vi "出厂检测.vi"() -> ()   [LabVIEW 2016]
uses:
  Ctl/AllSeting.ctl
  Ctl/Option.ctl
  controls/P2Judge QueueCtl.ctl
  <vilib>/vision/Image Controls.llb/IMAQ Image.ctl
panel:
  out "Array":u16[][](array[numeric])
  out "before substring":string
  out "Intensity Graph":u16[][](graph)
  out "Image":T1(plugin-control)
  in  "Button - Exit":bool
  in  "Button - Option":bool caption="Blank Button"
  in  "Button - Searchdata":bool caption="Blank Button"
  out "process":string
  in  "选项卡控件":enum32{"采集信息", "模组参数", "调试信息"}(tab)
  out "Tempparm_D合格？":bool
  out "NUC-T_D合格？":bool
  out "BT_D合格？":bool
  out "KT_D合格？":bool
  out "Tempparm合格？":bool
  out "NUC-T合格?":bool
  out "BT合格？":bool
  out "KT合格？":bool
  out "Tempparm一致性":bool
  out "NUC-T一致性":bool
  out "BT一致性":bool
  out "KT一致性":bool
  in  "固件版本":string
  in  "手动打印二维码":bool caption="Blank Button"
  in  "物料号":string="76"
  in  "型号":string(combo)="C"
  in  "打印列":u16(ring) items=["第一列", "第二列", "第三列", "第四列", "第五列"]
  in  "SN":string
  in  "PN":string
  out "盲元合格":bool
  in  "ID":string
  out "盲元数":dbl
  out "切换增益成功":bool
  out "state":string
  out "温度差值1":dbl
  out "读取温度1":dbl
  out "黑体设定温度1":dbl
  out "高增益温度误差在范围内":bool
  out "温度差值2":dbl
  out "读取温度2":dbl
  out "黑体设定温度2":dbl
  out "低增益温度误差在范围内":bool
  out "二维码信息":string
  out "当前流水号":string
  in  "当前增益模式":enum16{"低增益", "高增益"}(ring)
  out "近标靶是否合格":bool
  out "远标靶是否合格":bool
  out "近调焦垂直清晰度":dbl caption="垂直清晰度"
  out "近调焦水平清晰度":dbl caption="水平清晰度"
  out "远调焦水平清晰度":dbl caption="水平清晰度"
  out "远调焦垂直清晰度":dbl caption="垂直清晰度"
  out "低增益数据合格？":bool
  out "高增益数据合格？":bool
  out "Tempparam_Default":u8[](graph)
  out "NUC-T_Default":u16[](graph)
  out "BT_Default":i16[](graph)
  out "KT_Default":u16[](graph)
  out "Tempparam":u8[](graph)
  out "NUC-T":u16[](graph)
  out "BT":i16[](graph)
  out "KT":u16[](graph)
  in  "出图":bool
  out "Caldata.Fps":u16
  out "source path out":path
  out "调焦数值min":i32
  out "标定前盲元":dbl
  out "盲元表":dbl[][](array[numeric])
  out "调焦数值min2":i32
  out "检查锅盖竖纹是否合格":bool
  out "分辨率":string
  out "agc":u16
  in  "写入配置":bool caption="Blank Button"
  in  "打开AGC":bool caption="Blank Button"
  in  "读取盲元数":bool caption="Blank Button"
  in  "流水号归零":bool caption="Blank Button"
  in  "读ID":bool caption="Blank Button"
  in  "打快门":bool caption="Blank Button"
  out "参数存储地址":path
  out "Numeric":dbl format="%#_13g"
  in  "Button - start":bool caption="Blank Button"
  in  "完成":bool caption="Blank Button"
  # "在存储地址放入模板"
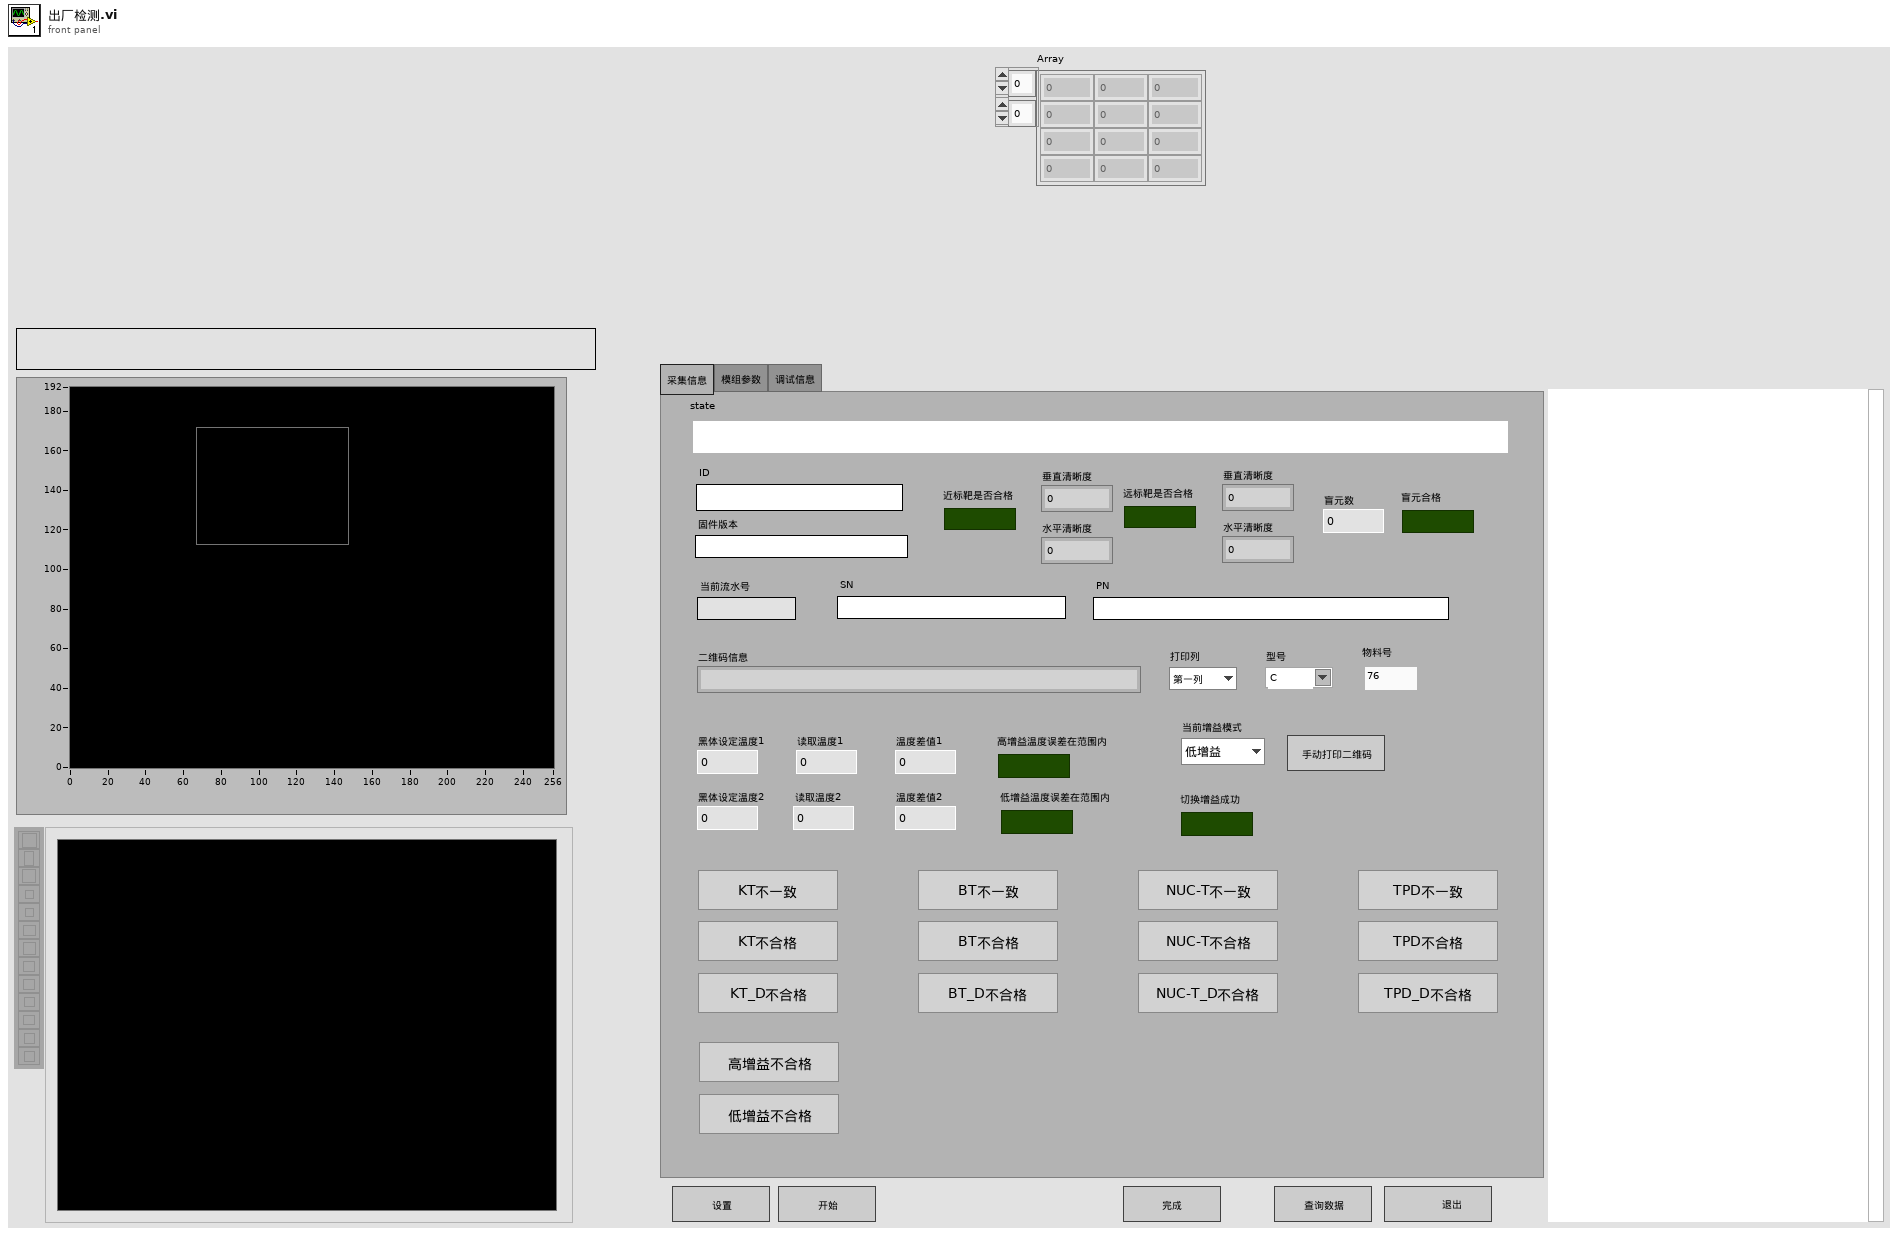
[diagram p1: front panel]
types:
  T1 = typedef "IMAQ Image.ctl" = refnum<image>
  T2 = typedef "AllSeting.ctl" = cluster{"Caldata":T3}
  T3 = typedef "Option.ctl" = cluster{"分辨率":string, "Fps":u16, "工单号":string, "操作人":string, "增益模式":enum16{"高低增益切换", "高增益"}, "黑体设定温度1":dbl, "温差范围1":dbl, "出图到测温等待时间":dbl, "调焦数值min":i32, "盲元阈值":dbl, "盲元采样帧数":u16, "调焦数值min2":i32, "黑体设定温度2":dbl, "温差范围2":dbl, "ID选择":enum16{"旧ID", "新ID"}, "快门时间间隔设置":cluster{"快门第一次延时时间":u16, "快门第二次延时时间":u16, "切换增益后快门第一次延时时间":u16, "切换增益后快门第二次延时时间":u16}, "产品名":string, "镜头":string, "测温功能":string, "产品料号":string, "打印机VISA":refnum<visa-resource-name>, "焦距选择":enum32{"Radio Selection 1", "Radio Selection 2", "Radio Selection 3"}, "工位":string, "服务器保存地址":path}
  T4 = typedef "P2Judge QueueCtl.ctl" = enum16{"Main", "Device", "Picture"}
  T5 = typedef "QueueModeCtl.ctl" = enum16{"<no operate>", "Send", "Send(head)", "Flush", "Destory", "Send>All", "Send>All(head)", "Flush All", "Destory All"}
  T6 = cluster{"CalData":path, "Datasave":path, "Data":path}
  T7 = enum32{"Radio Selection 1", "Radio Selection 2", "Radio Selection 3"}
  T8 = cluster{"快门第一次延时时间":u16, "快门第二次延时时间":u16, "切换增益后快门第一次延时时间":u16, "切换增益后快门第二次延时时间":u16}
  T9 = typedef "LVPointDoubleTypeDef.ctl" = cluster{"Cursor X":dbl, "Cursor Y":dbl}
  T10 = enum32{"invalid app kind", "Development System", "Run Time System", "Student Edition", "Embedded LabVIEW", "Evaluation", "Custom"}
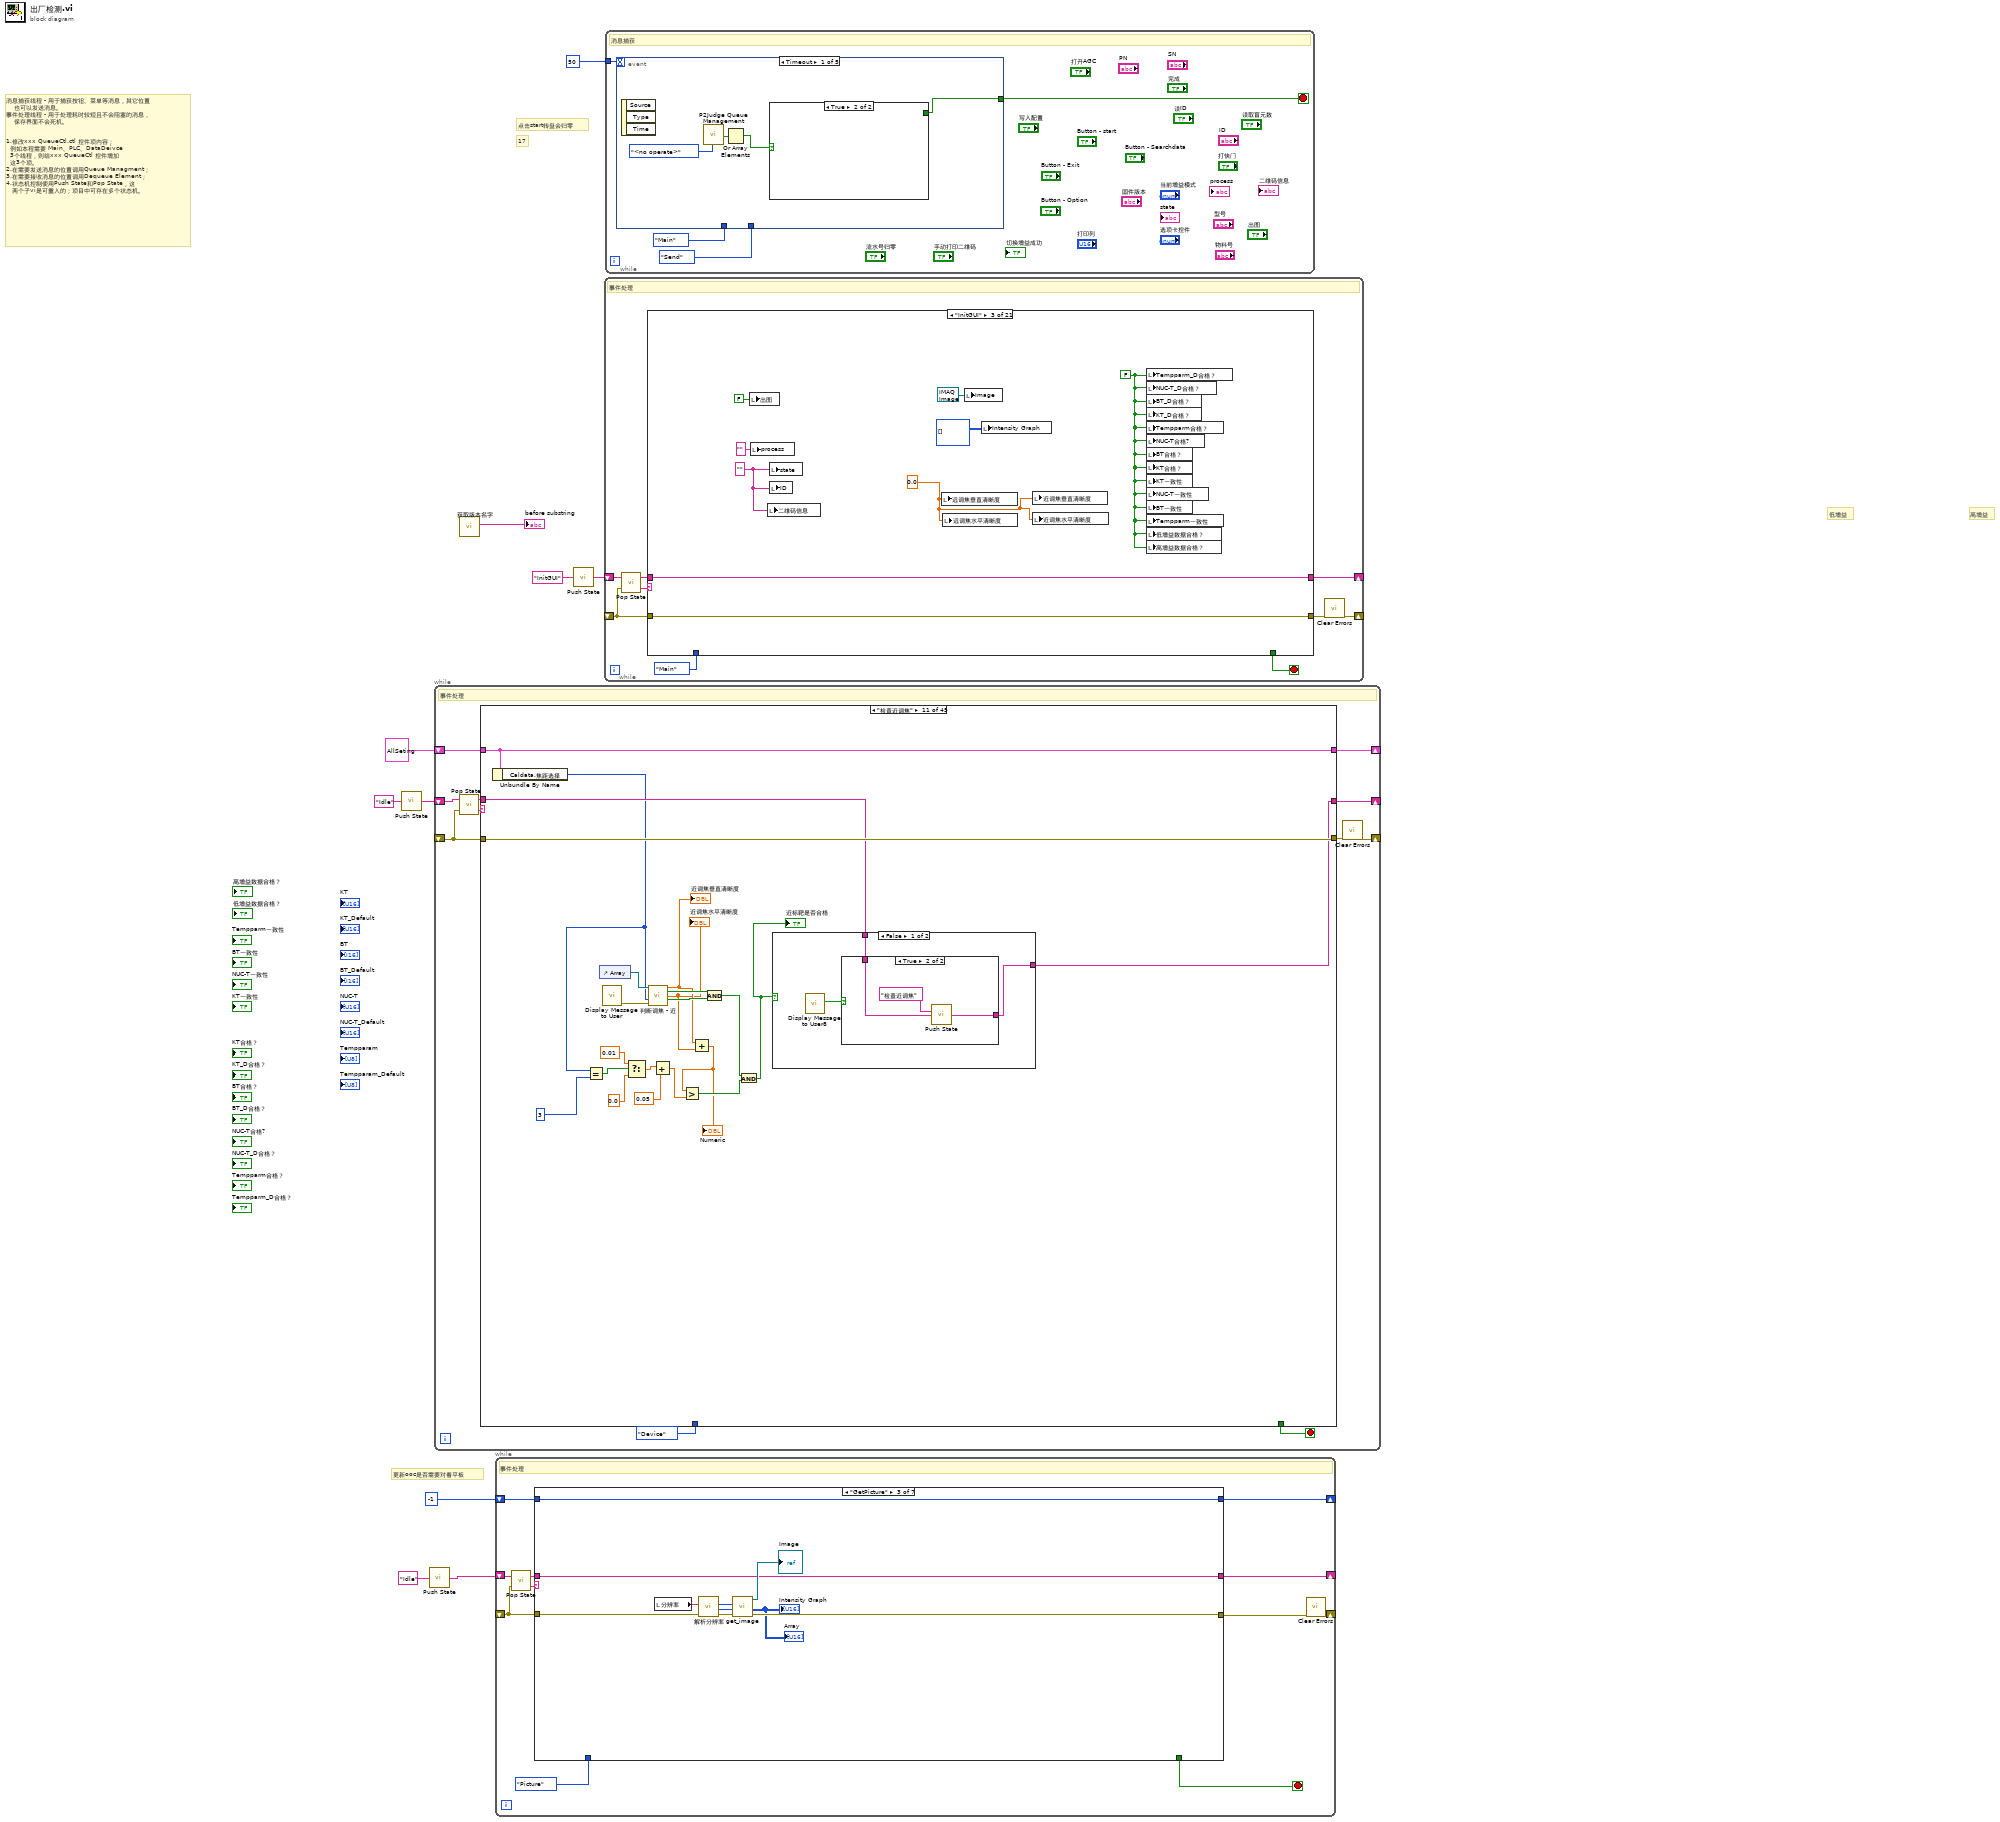
[diagram p0: block diagram]
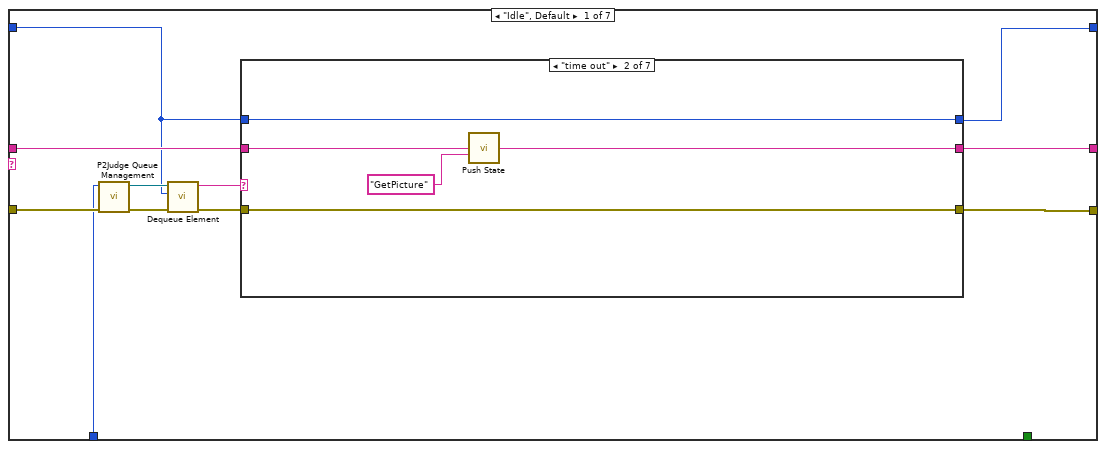
[diagram p2: hidden frame]
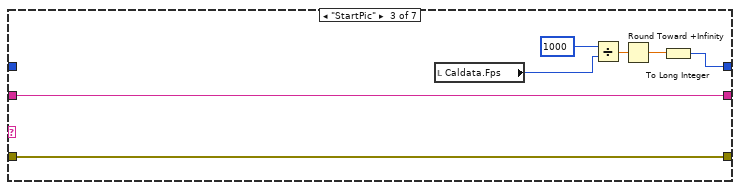
[diagram p4: hidden frame]
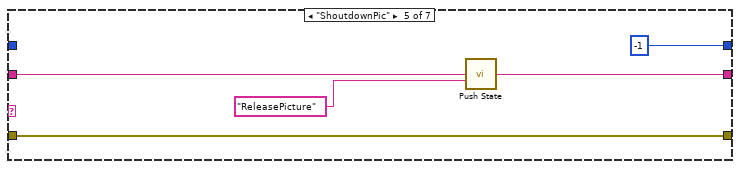
[diagram p6: hidden frame]
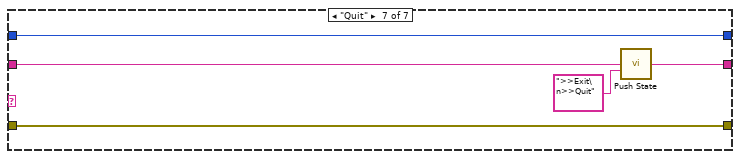
[diagram p8: hidden frame]
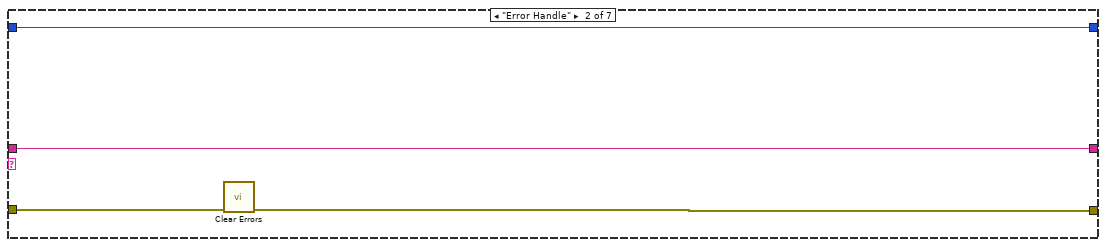
[diagram p9: hidden frame]
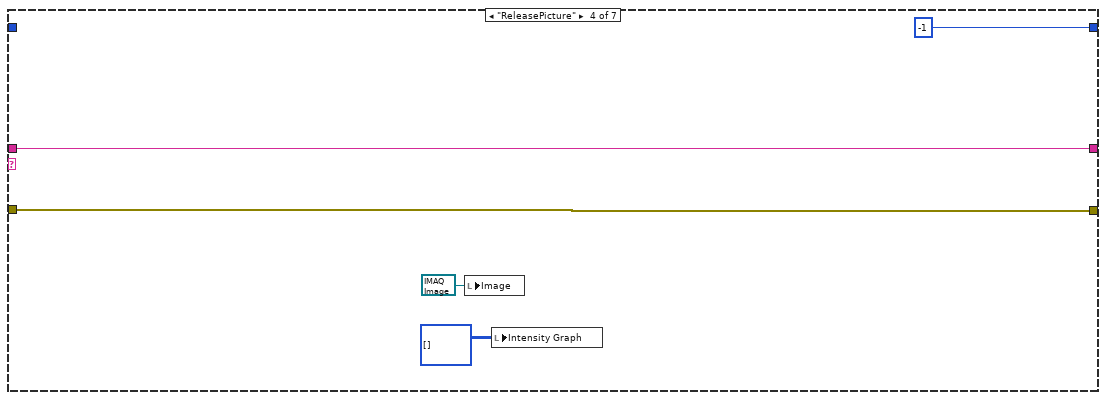
[diagram p10: hidden frame]
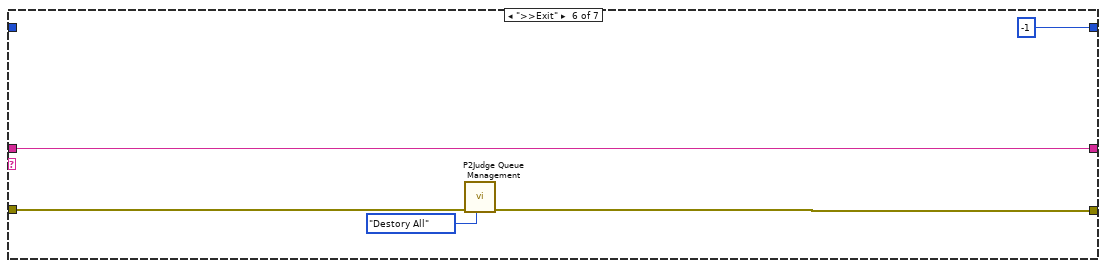
[diagram p12: hidden frame]
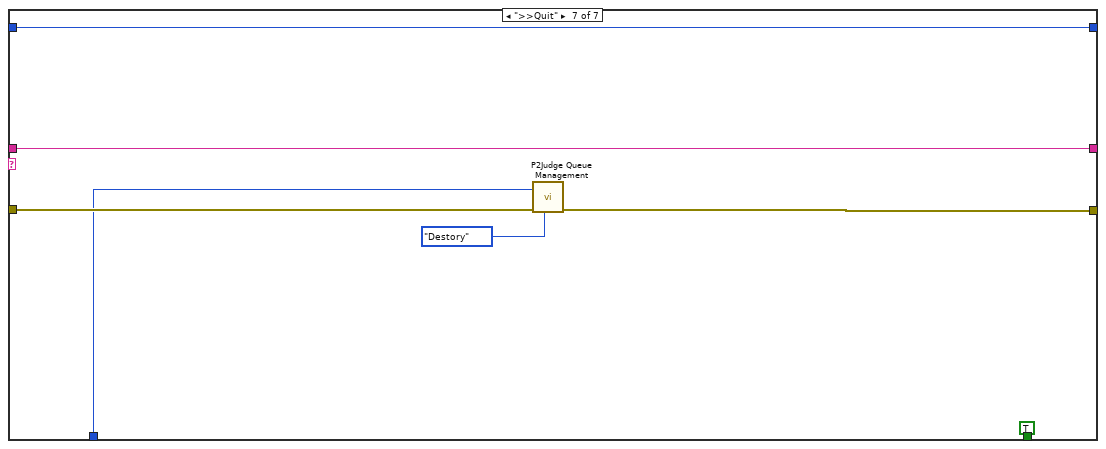
[diagram p13: hidden frame]
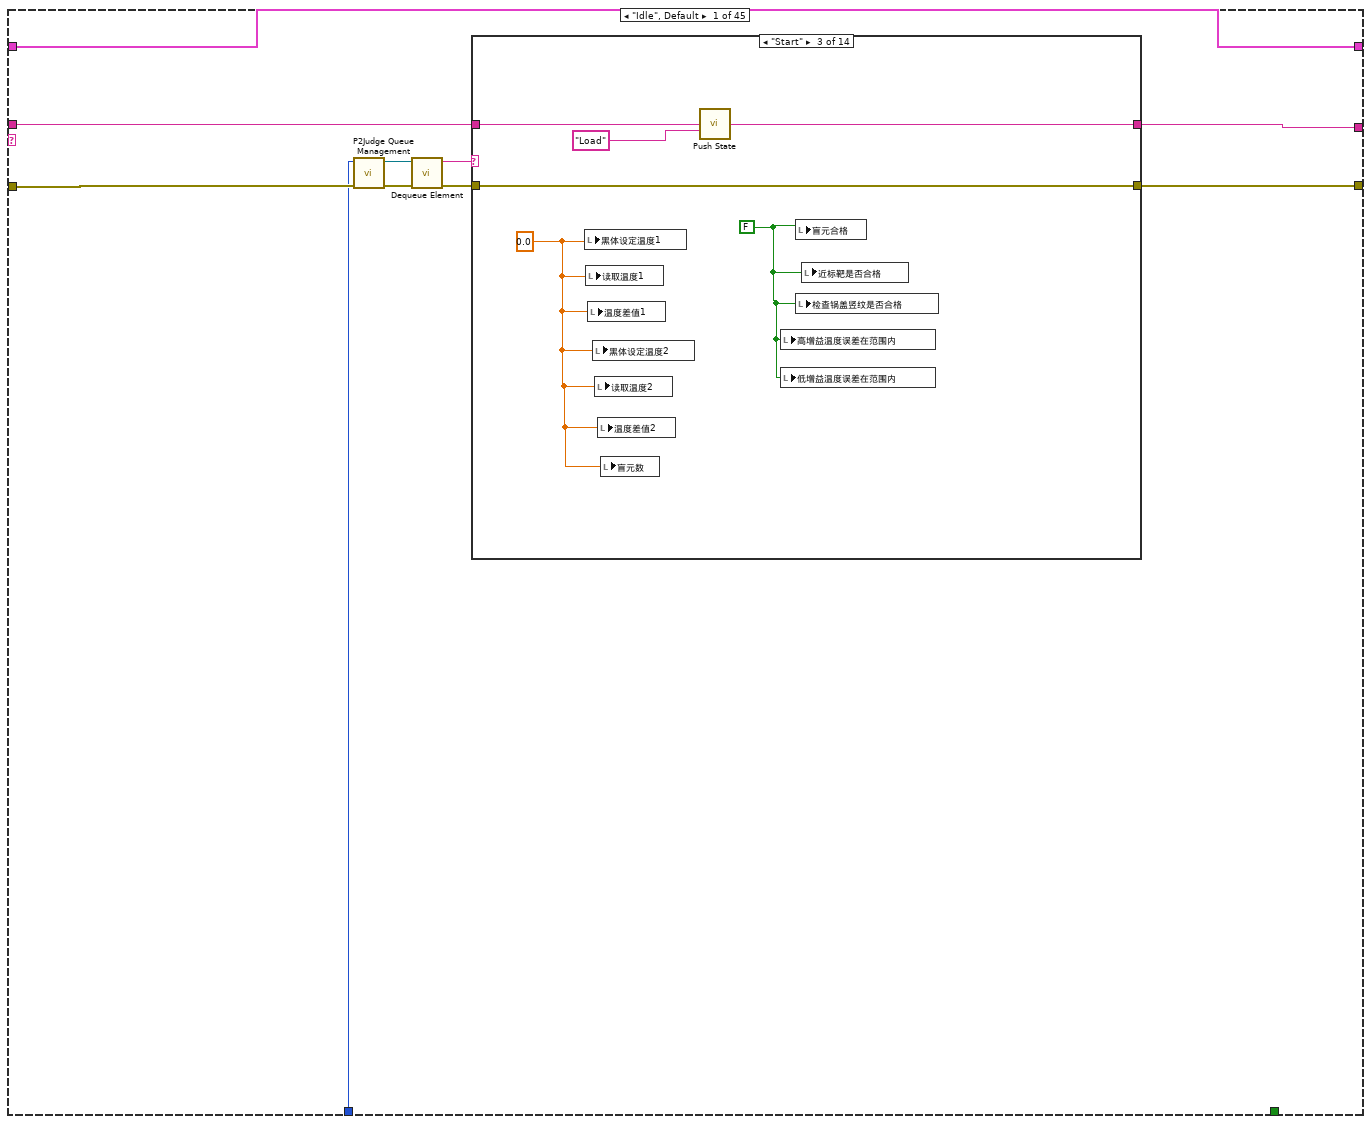
[diagram p14: hidden frame]
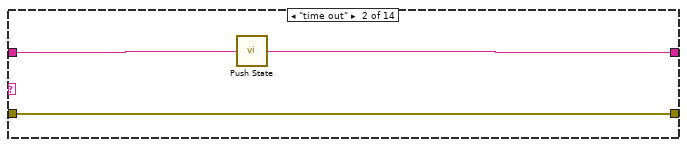
[diagram p16: hidden frame]
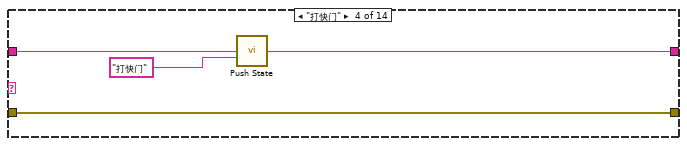
[diagram p17: hidden frame]
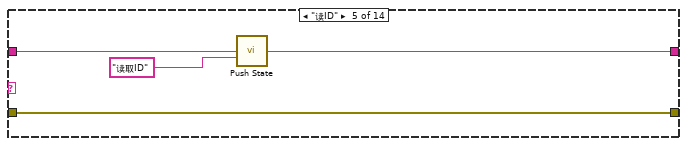
[diagram p18: hidden frame]
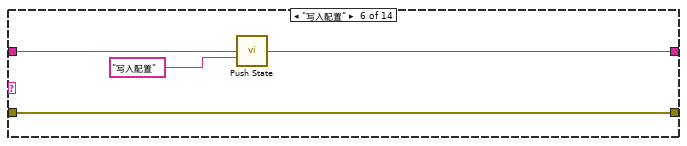
[diagram p19: hidden frame]
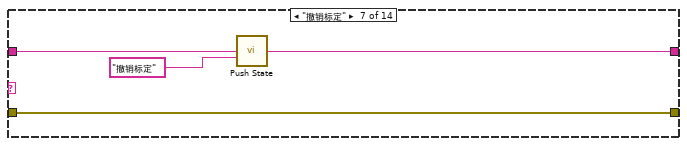
[diagram p20: hidden frame]
diagram:
  # "高增益"
  # "低增益"
  # "17"
  # "更新ooc是否需要对着平板"
  # "点击start转盘会归零"
  # "消息捕获线程 - 用于捕获按钮、菜单等消息，其它位置\n    也可以发送消息。\n事件处理线程 - 用于处理耗时较短且不会阻塞的消息，\n    保存界面不会死机。\n\n\n1.修改xxx QueueCtl.ctl 控件项内容；\n  例如本程需要 Main、PLC、DataDeivce\n  3个线程，则给xxx QueueCtl 控件增加\n  这3个项。\n2.在需要发送消息的位置调用Queue Managment；\n3.在需要接收消息的位置调用Dequeue Element；\n4.状态机控制使用Push State和Pop State，这\n   两个子vi是可重入的；项目中可存在多个状态机。"
  n1 = call "Push State.vi"("States In"="Idle") -> ("States Out"=w6:string)  [unwired: 14 in]
  n2 = call "Push State.vi"("States In"="Idle") -> ("States Out"=w3:string)  [unwired: 14 in]
  n3 = while {
    shift-right: [w19] -> _
    shift-left: w6 -> [w21]
    shift-right: [w11] -> _
    shift-left: _ -> [w17]
    shift-right: [w14] -> _
    shift-left: T2 {"Caldata"={"分辨率"="", "Fps"=0, "工单号"="", "操作人"="", "增益模式"=enum."高低增益切换", "黑体设定温度1"=0.0, "温差范围1"=0.0, "出图到测温等待时间"=0.0, "调焦数值min"=0, "盲元阈值"=0.0, "盲元采样帧数"=0, "调焦数值min2"=0, "黑体设定温度2"=0.0, "温差范围2"=0.0, "ID选择"=enum."旧ID", "快门时间间隔设置"={"快门第一次延时时间"=200, "快门第二次延时时间"=200, "切换增益后快门第一次延时时间"=200, "切换增益后快门第二次延时时间"=200}, "产品名"="Tiny1-C", "镜头"="02011X", "测温功能"="WR", "产品料号"="", "打印机VISA"="", "焦距选择"=enum."Radio Selection 1", "工位"="0001", "服务器保存地址"=path ""}} ("all setting") -> [w13]
    stop <- w16 stop-if-true
    # "事件处理"
    n4 = call "Pop State.vi"("error in (no error)"=w17, "Pre States"=w21) -> ("New State"=w20:string, "Remaining States"=w18:string)
    n5 = case shown="\"检查近调焦\"" w20 {
      tunnel: [w25 w88 w91 w112 w141 w171 w205 w232 w252 w265 w292 w333 w350 w358 w400 w438 w453 w484 w506 w525 w574 w625 w650 w678 w694 w706 w766 w786 w881 w1045 w1080 w1102 w1109 w1145 w1167 w1244 w1303 w1350 w1383 w1411 w1413 w1437 w1447 w1475 w1482] -> w19
      tunnel: w18 -> [w24 w88 w91 _ w143 w172 w207 w234 w252 w265 w291 w332 w350 w355 w401 w439 w454 w485 w507 w526 w575 w626 w651 w675 w694 w706 w767 w788 w882 w1046 w1081 w1102 w1110 w1145 w1168 w1245 w1304 w1351 w1384 w1411 w1414 w1437 w1448 w1475 w1482]
      tunnel: [w28 w86 w90 w117 w144 w164 w206 w233 w253 w266 w295 w336 w347 w359 w402 w440 w455 w486 w508 w527 w576 w627 w652 w679 w695 w705 w768 w846 w880 w1047 w1082 w1101 w1111 w1140 w1169 w1246 w1288 w1334 w1382 w1409 w1415 w1438 w1449 w1473 w1478] -> w12
      tunnel: w17 -> [w31 w87 w90 w122 w140 w167 w211 w238 w257 w270 w295 w336 w348 w368 w395 w433 w460 w488 w510 w528 w577 w628 w653 w680 w700 w708 w771 w847 w941 w1048 w1085 w1103 w1116 w1146 w1173 w1248 w1305 w1352 w1388 w1410 w1419 w1441 w1453 w1474 w1479]
      tunnel: [_ _ _ _ _ _ _ _ _ _ _ _ _ _ _ _ _ _ _ _ _ _ _ _ _ _ _ _ _ _ _ _ _ _ _ _ _ _ _ _ _ _ _ _ TRUE] -> w16
      tunnel: P2Judge_QueueCtl."Device" ("Queue Index") -> [w23 _ _ _ _ _ _ _ _ _ _ _ _ _ _ _ _ _ _ _ _ _ _ _ _ _ _ _ _ _ _ _ _ _ _ _ _ _ _ _ _ _ _ _ w1477]
      tunnel: [w22 w85 w89 w114 w130 w163 w215 w239 w251 w264 w289 w330 w349 w370 w403 w441 w465 w475 w503 w524 w573 w624 w649 w677 w699 w707 w776 w844 w940 w1040 w1090 w1108 w1121 w1139 w1158 w1242 w1299 w1346 w1393 w1408 w1412 w1440 w1451 w1471 w1476] -> w14
      tunnel: w13 -> [w22 w85 w89 w113 w130 w163 w215 w239 w251 w264 w289 w330 w349 w370 w403 w441 w465 w475 w503 w524 w573 w624 w649 w677 w699 w707 w776 w844 w940 w1040 w1090 w1108 w1121 w1139 w1158 w1242 w1299 w1346 w1393 w1408 w1412 w1440 w1451 w1471 w1476]
      frame "Idle", Default {
        n6 = call "P2Judge Queue Management.vi"("error in"=w31, "Queue Index"=w23) -> ("error out"=w30:errorcluster, "Queue"=w29:refnum<queue>)  [unwired: 7 in, 1 out]
        n7 = call "Dequeue Element.vi"("error in"=w30, "Queue"=w29) -> ("error out"=w27:errorcluster, "Command"=w26:string)  [unwired: 7 in, 1 out]
        n8 = case shown="\"Start\"" w26 {
          tunnel: [w33 w36 w42 w46 w50 w54 w58 w62 w66 w70 w74 w78 w80 w84] -> w28
          tunnel: w27 -> [w33 w36 w42 w46 w50 w54 w58 w62 w66 w70 w74 w78 w80 w84]
          tunnel: [w32 w34 w40 w44 w48 w52 w56 w60 w64 w68 w72 w76 w79 w82] -> w25
          tunnel: w24 -> [w32 w35 w41 w45 w49 w53 w57 w61 w65 w69 w73 w77 w79 w83]
          frame Default {
          }
          frame "time out" {
            n9 = call "Push State.vi"("States In"=w35) -> ("States Out"=w34:string)  [unwired: 14 in]
          }
          frame "Start" {
            w38 = 0.0
            w37 = FALSE
            n10 = local write "黑体设定温度1"(w38) -> ()
            n11 = local write "读取温度1"(w38) -> ()
            n12 = local write "温度差值1"(w38) -> ()
            n13 = local write "黑体设定温度2"(w38) -> ()
            n14 = local write "读取温度2"(w38) -> ()
            n15 = local write "温度差值2"(w38) -> ()
            n16 = local write "盲元数"(w38) -> ()
            n17 = call "Push State.vi"("States In"=w41, "States End"="Load") -> ("States Out"=w40:string)  [unwired: 13 in]
            n18 = local write "高增益温度误差在范围内"(w37) -> ()
            n19 = local write "低增益温度误差在范围内"(w37) -> ()
            n20 = local write "盲元合格"(w37) -> ()
            n21 = local write "检查锅盖竖纹是否合格"(w37) -> ()
            n22 = local write "近标靶是否合格"(w37) -> ()
          }
          frame "打快门" {
            n23 = call "Push State.vi"("States In"=w45, "States End"="打快门") -> ("States Out"=w44:string)  [unwired: 13 in]
          }
          frame "读ID" {
            n24 = call "Push State.vi"("States In"=w49, "States End"="读取ID") -> ("States Out"=w48:string)  [unwired: 13 in]
          }
          frame "写入配置" {
            n25 = call "Push State.vi"("States In"=w53, "States End"="写入配置") -> ("States Out"=w52:string)  [unwired: 13 in]
          }
          frame "撤销标定" {
            n26 = call "Push State.vi"("States In"=w57, "States End"="撤销标定") -> ("States Out"=w56:string)  [unwired: 13 in]
          }
          frame "打开AGC" {
            n27 = call "Push State.vi"("States In"=w61, "States End"="打开AGC") -> ("States Out"=w60:string)  [unwired: 13 in]
          }
          frame "打印二维码" {
            n28 = call "Push State.vi"("States In"=w65, "States End"="打印二维码") -> ("States Out"=w64:string)  [unwired: 13 in]
          }
          frame "流水号归零" {
            n29 = call "Push State.vi"("States In"=w69, "States End"="流水号归零") -> ("States Out"=w68:string)  [unwired: 13 in]
          }
          frame "读取盲元数" {
            n30 = call "Push State.vi"("States In"=w73, "States End"="读取盲元数") -> ("States Out"=w72:string)  [unwired: 13 in]
          }
          frame "完成" {
            n31 = call "Push State.vi"("States In"=w77, "States End"="保存出厂检测数据\n关闭相机") -> ("States Out"=w76:string)  [unwired: 13 in]
          }
          frame "error" {
          }
          frame "Quit" {
            n32 = call "Push State.vi"("States In"=w83, "States End"=">>Exit\n>>Quit" ("Remaining States")) -> ("States Out"=w82:string)  [unwired: 13 in]
          }
        }
      }
      frame "Error Handle" {
        n33 = call <vilib>:"Clear Errors.vi"("error in (no error)"=w87) -> ("error out"=w86:errorcluster)  [unwired: 5 in, 1 out]
      }
      frame ">>Init" {
      }
      frame "Load" {
        w92 = FALSE ("Tempparm_D合格？")
        w124 = "下载配置" ("state")
        n34 = local read "process"() -> (w125:string)
        n35 = property on="state" class="Str"(error in=w122, "Value"=w124) -> (error out=w126:errorcluster)  [unwired: 1 in, 1 out]
        n36 = call "process.vi"("error in"=w126, "state"=w124, "process in"=w125) -> ("error out"=w121:errorcluster, "process out"=w123:string)  [unwired: 7 in]
        n37 = local write "Tempparm_D合格？"(w92) -> ()
        n38 = local write "NUC-T_D合格？"(w92) -> ()
        n39 = local write "BT_D合格？"(w92) -> ()
        n40 = local write "KT_D合格？"(w92) -> ()
        n41 = local write "Tempparm合格？"(w92) -> ()
        n42 = local write "NUC-T合格?"(w92) -> ()
        n43 = local write "BT合格？"(w92) -> ()
        n44 = local write "KT合格？"(w92) -> ()
        n45 = local write "KT一致性"(w92) -> ()
        n46 = local write "NUC-T一致性"(w92) -> ()
        n47 = local write "BT一致性"(w92) -> ()
        n48 = local write "Tempparm一致性"(w92) -> ()
        n49 = local write "低增益数据合格？"(w92) -> ()
        n50 = local write "高增益数据合格？"(w92) -> ()
        n51 = call "Path.vi"() -> ("path"=w120:T6)  [unwired: 9 in]
        n52 = local write "process"(w123) -> ()
        n53 = Unbundle By Name(w120) -> ("CalData"=w119:path)
        n54 = call "Path.vi"() -> ()  [unwired: 9 in, 1 out]
        n55 = call "loadorsave_Option.vi"("save?"=FALSE, "error in"=w121, "Path in"=w119) -> ("error out"=w118:errorcluster, "Caldata out"=w115:T3)  [unwired: 6 in, 1 out]
        n56 = Unbundle By Name(w115) -> ("调焦数值min2"=→"调焦数值min2":i32, "调焦数值min"=→"调焦数值min":i32, "工单号"=w116:string, "增益模式"=w107:enum16{"高低增益切换", "高增益"}, "分辨率"=w100:string, "服务器保存地址"=w94:path)
        "分辨率" <- w100
        n57 = case shown="\"高低增益切换\", Default" w107 {
          tunnel: ["打开相机\n计算流水号\n读取ID\n读取固件版本\n关闭AGC\n关闭自动快门\n切换出图为SNR\n切换低增益\n出图到测温等待时间\n打快门\n读取低增益温度\n切换高增益\n出图到测温等待时间\n打快门\n读取高增益温度\n打快门\n检查近调焦\n检查远调焦\n检查锅盖竖纹\n打快门\n读取标定盲元\n打开自动快门\n绑定ID\n写入SN\n写入PN\n读取SNPN\n打开AGC\n保存数据\n生成出厂配置\n检查模组高增益参数\n检查模组低增益参数\n打印二维码\n出厂检完成" "打开相机\n计算流水号\n读取ID\n读取固件版本\n读取SNPN\n关闭AGC\n关闭自动快门\n切换出图为SNR\n切换高增益\n出图到测温等待时间\n打快门\n读取高增益温度\n打快门\n检查近调焦\n检查远调焦\n检查锅盖竖纹\n打快门\n读取标定盲元\n打开自动快门\n绑定ID\n写入SN\n写入PN\n读取SNPN\n打开AGC\n保存数据\n生成出厂配置\n检查模组高增益参数\n打印二维码\n出厂检完成"] -> w112
          frame "高低增益切换", Default {
          }
          frame "高增益" {
          }
        }
        n58 = Equal?(x=w100, y="256*192") -> (x = y?=w96:bool)
        n59 = Select(t="Tiny1Cflash.xlsx", s=w96, f="Tiny1Cflash小分辨率.xlsx") -> (s? t:f=w95:string)
        n60 = call "复制模板.vi"("error in"=w118, "服务器地址"=w94, "工单号"=w116) -> ("error out"=w109:errorcluster, "参数存储地址"=→"参数存储地址":path, "source path out"=→"source path out":path)  [unwired: 6 in]
        n61 = call "Path.vi"() -> ("path"=w106:T6)  [unwired: 9 in]
        n62 = Unbundle By Name(w106) -> ("Data"=w105:path)
        n63 = Build Path(base path=w105, name or relative path=w95) -> (appended path=w104:path)
        n64 = call "Read_Address_Map.vi"("file path"=w104) -> ("error out"=w103:errorcluster, "all rows"=w102:string[][])  [unwired: 9 in]
        n65 = Bundle By Name(cluster=w113, "Caldata"=w115) -> (w114:T2)
        n66 = call "2DStrArrayToEle.vi"("Mothed"=enum16{"init", "Get", "Set", "Close"}."Set", "error in"=w103, "all rows"=w102) -> ()  [unwired: 5 in, 4 out]
        n67 = call <vilib>:"Clear Errors.vi"("error in (no error)"=w109) -> ("error out"=w117:errorcluster)  [unwired: 5 in, 1 out]
      }
      frame "打开相机" {
        w138 = "打开相机" ("state")
        n68 = local read "process"() -> (w137:string)
        n69 = property on="state" class="Str"(error in=w140, "Value"=w138) -> (error out=w136:errorcluster)  [unwired: 1 in, 1 out]
        n70 = call "process.vi"("error in"=w136, "state"=w138, "process in"=w137) -> ("error out"=w135:errorcluster, "process out"=w139:string)  [unwired: 7 in]
        n71 = local write "process"(w139) -> ()
        n72 = Unbundle By Name(w130) -> ("Caldata.分辨率"=w134:string, "Caldata.Fps"=w133:u16)
        "Caldata.Fps" <- w133
        n73 = call "打开相机.vi"("error in"=w135, "FPS"=w133, "分辨率"=w134) -> ("error out"=w131:errorcluster, "result"=w132:bool)  [unwired: 6 in, 1 out]
        n74 = case shown="True" w132 {
          tunnel: ["操作失败关闭相机" w150] -> w142
          tunnel: w131 -> [w145 w149]
          tunnel: [w145 w147] -> w144
          tunnel: w143 -> [_ w150]
          frame False {
          }
          frame True {
            n75 = property on="出图" class="Bool (strict)"(error in=w149, "Val(Sgnl)"=TRUE ("Value (Signaling)")) -> (error out=w147:errorcluster)  [unwired: 1 in, 1 out]
          }
        }
        n76 = call "Push State.vi"("States In"=w142) -> ("States Out"=w141:string)  [unwired: 14 in]
      }
      frame "读取ID" {
        w170 = "读取ID" ("state")
        w176 = "_"
        n77 = local read "process"() -> (w169:string)
        n78 = property on="state" class="Str"(error in=w167, "Value"=w170) -> (error out=w168:errorcluster)  [unwired: 1 in, 1 out]
        n79 = call "process.vi"("error in"=w168, "state"=w170, "process in"=w169) -> ("error out"=w166:errorcluster, "process out"=w165:string)  [unwired: 7 in]
        n80 = local write "process"(w165) -> ()
        n81 = call "ReadID.vi"("error in"=w166) -> ("error out"=w173:errorcluster, "data out"=w189:u8[], "return"=w175:i32)  [unwired: 8 in]
        n82 = Index Array(array=w189) -> (element #1=w188:u8, element #2=w187:u8, element #3=w186:u8, element #4=w185:u8, element #5=w184:u8, element #6=w183:u8, element #7=w162:u8, element #8=w161:u8, element #9=w160:u8, element #10=w159:u8)  [unwired: 10 in]
        n83 = Join Numbers(hi=w160, lo=w159) -> ((hi.lo)=w157:u16)
        n84 = Join Numbers(hi=w162, lo=w161) -> ((hi.lo)=w158:u16)
        n85 = Join Numbers(hi=w188, lo=w187) -> ((hi.lo)=w182:u16)
        n86 = Join Numbers(hi=w186, lo=w185) -> ((hi.lo)=w181:u16)
        n87 = Join Numbers(hi=w184, lo=w183) -> ((hi.lo)=w180:u16)
        n88 = Join Numbers(hi=w158, lo=w157) -> ((hi.lo)=w156:u32)
        n89 = Number To Decimal String(number=w156) -> (decimal integer string=w153:string)  [unwired: 1 in]
        n90 = Number To Decimal String(number=w180) -> (decimal integer string=w177:string)  [unwired: 1 in]
        n91 = Number To Decimal String(number=w182) -> (decimal integer string=w179:string)  [unwired: 1 in]
        n92 = Number To Decimal String(number=w181) -> (decimal integer string=w178:string)  [unwired: 1 in]
        n93 = Unbundle By Name(w163) -> ("Caldata.ID选择"=w155:enum16{"旧ID", "新ID"})
        n94 = Concatenate Strings(w179, w176, w178, w176, w177) -> (w154:string)
        n95 = Equal To 0?(x=w155) -> (x = 0?=w152:bool)
        n96 = Select(t=w154, s=w152, f=w153) -> (s? t:f=w151:string)
        n97 = local write "ID"(w151) -> ()
        n98 = Equal To 0?(x=w175) -> (x = 0?=w174:bool)
        n99 = case shown="True" w174 {
          tunnel: w173 -> [w191 w193]
          tunnel: [w191 w192] -> w164
          tunnel: w172 -> [_ w198]
          tunnel: ["操作失败关闭相机" w198] -> w171
          frame False {
          }
          frame True {
            w194 = "读取ID成功" ("state")
            n100 = local read "process"() -> (w195:string)
            n101 = property on="state" class="Str"(error in=w193, "Value"=w194) -> (error out=w196:errorcluster)  [unwired: 1 in, 1 out]
            n102 = call "process.vi"("error in"=w196, "state"=w194, "process in"=w195) -> ("error out"=w192:errorcluster, "process out"=w197:string)  [unwired: 7 in]
            n103 = local write "process"(w197) -> ()
          }
        }
      }
      frame "关闭AGC" {
        w214 = "关闭AGC" ("state")
        n104 = local read "process"() -> (w213:string)
        n105 = property on="state" class="Str"(error in=w211, "Value"=w214) -> (error out=w212:errorcluster)  [unwired: 1 in, 1 out]
        n106 = call "process.vi"("error in"=w212, "state"=w214, "process in"=w213) -> ("error out"=w200:errorcluster, "process out"=w210:string)  [unwired: 7 in]
        n107 = local write "process"(w210) -> ()
        n108 = call "读取AGC.vi"("error in (no error)"=w200) -> ("error out"=w199:errorcluster, "(hi.lo)"=→"agc":u16)  [unwired: 9 in]
        n109 = call "关闭AGC.vi"("error in"=w199) -> ("error out"=w204:errorcluster, "return"=w209:i32)  [unwired: 9 in]
        n110 = Equal To 0?(x=w209) -> (x = 0?=w208:bool)
        n111 = call "Wait (ms)__ogtk.vi"("error in (no error)"=w204, "milliseconds to wait"=u32 1000) -> ("error out"=w203:errorcluster)  [unwired: 8 in, 1 out]
        n112 = case shown="True" w208 {
          tunnel: w207 -> [_ w224]
          tunnel: ["操作失败关闭相机" w224] -> w205
          tunnel: w203 -> [w216 w219]
          tunnel: [w216 w218] -> w206
          frame False {
          }
          frame True {
            w221 = "关闭AGC成功" ("state")
            n113 = local read "process"() -> (w222:string)
            n114 = property on="state" class="Str"(error in=w219, "Value"=w221) -> (error out=w223:errorcluster)  [unwired: 1 in, 1 out]
            n115 = call "process.vi"("error in"=w223, "state"=w221, "process in"=w222) -> ("error out"=w218:errorcluster, "process out"=w220:string)  [unwired: 7 in]
            n116 = local write "process"(w220) -> ()
          }
        }
      }
      frame "打开AGC" {
        w229 = "打开AGC" ("state")
        n117 = local read "process"() -> (w227:string)
        n118 = property on="state" class="Str"(error in=w238, "Value"=w229) -> (error out=w231:errorcluster)  [unwired: 1 in, 1 out]
        n119 = call "process.vi"("error in"=w231, "state"=w229, "process in"=w227) -> ("error out"=w230:errorcluster, "process out"=w228:string)  [unwired: 7 in]
        n120 = local write "process"(w228) -> ()
        n121 = local read "agc"() -> (w226:u16)
        n122 = To Unsigned Long Integer(number=w226) -> (unsigned 32bit integer=w225:u32)
        n123 = call "打开AGC.vi"("error in"=w230, "dwAddr1"=w225) -> ("error out"=w236:errorcluster, "return"=w237:i32)  [unwired: 8 in]
        n124 = Equal To 0?(x=w237) -> (x = 0?=w235:bool)
        n125 = case shown="True" w235 {
          tunnel: w234 -> [_ w248]
          tunnel: ["操作失败关闭相机" w248] -> w232
          tunnel: w236 -> [w240 w243]
          tunnel: [w240 w242] -> w233
          frame False {
          }
          frame True {
            w245 = "打开AGC成功" ("state")
            n126 = local read "process"() -> (w246:string)
            n127 = property on="state" class="Str"(error in=w243, "Value"=w245) -> (error out=w247:errorcluster)  [unwired: 1 in, 1 out]
            n128 = call "process.vi"("error in"=w247, "state"=w245, "process in"=w246) -> ("error out"=w242:errorcluster, "process out"=w244:string)  [unwired: 7 in]
            n129 = local write "process"(w244) -> ()
          }
        }
      }
      frame "切换出图为SNR" {
        w250 = 0
        w261 = "切换出图为SNR" ("state")
        n130 = local read "process"() -> (w260:string)
        n131 = property on="state" class="Str"(error in=w257, "Value"=w261) -> (error out=w259:errorcluster)  [unwired: 1 in, 1 out]
        n132 = call "process.vi"("error in"=w259, "state"=w261, "process in"=w260) -> ("error out"=w256:errorcluster, "process out"=w258:string)  [unwired: 7 in]
        n133 = local write "process"(w258) -> ()
        n134 = local read "分辨率"() -> (w249:string)
        n135 = call "Preview STOP.vi"("error in"=w256, "preview path"=w250) -> ("error out"=w255:errorcluster)  [unwired: 8 in, 1 out]
        n136 = call "Preview Start.vi"("error in"=w255, "分辨率"=w249, "preview path"=w250) -> ("error out"=w254:errorcluster)  [unwired: 7 in, 1 out]
        n137 = call "切换出图为SNR.vi"("error in"=w254) -> ("error out"=w253:errorcluster)  [unwired: 9 in, 1 out]
      }
      frame "切换出图为TNR" {
        w263 = 0
        w274 = "切换出图为SNR" ("state")
        n138 = local read "process"() -> (w273:string)
        n139 = property on="state" class="Str"(error in=w270, "Value"=w274) -> (error out=w272:errorcluster)  [unwired: 1 in, 1 out]
        n140 = call "process.vi"("error in"=w272, "state"=w274, "process in"=w273) -> ("error out"=w269:errorcluster, "process out"=w271:string)  [unwired: 7 in]
        n141 = local write "process"(w271) -> ()
        n142 = local read "分辨率"() -> (w262:string)
        n143 = call "Preview STOP.vi"("error in"=w269, "preview path"=w263) -> ("error out"=w268:errorcluster)  [unwired: 8 in, 1 out]
        n144 = call "Preview Start.vi"("error in"=w268, "分辨率"=w262, "preview path"=w263) -> ("error out"=w267:errorcluster)  [unwired: 7 in, 1 out]
        n145 = call "切换出图为TNR.vi"("error in"=w267) -> ("error out"=w266:errorcluster)  [unwired: 9 in, 1 out]
      }
      frame "检查近调焦" {
        n146 = Unbundle By Name(w289) -> ("Caldata.焦距选择"=w283:T7)
        n147 = Equal?(x=w283, y=3) -> (x = y?=w281:bool)
        n148 = control-ref of="Array"() -> (w296:refnum<vi>)
        n149 = call "Display Message to User"() -> ("error out"=w290:errorcluster)  [unwired: 10 in, 1 out]
        n150 = Select(t=0.01, s=w281, f=0.0) -> (s? t:f=w278:dbl)
        n151 = call "判断调焦 - 近.vi"("Arr Refnum"=w296, "选项"=w283, "error in"=w290) -> ("垂直清晰度-数值"=w288:dbl, "垂直清晰度"=w294:bool, "水平清晰度-数值"=w287:dbl, "水平清晰度"=w293:bool)  [unwired: 8 in, 1 out]
        "近调焦垂直清晰度" <- w288
        "近调焦水平清晰度" <- w287
        n152 = Add(x=w278, y=0.05) -> (x+y=w276:dbl)
        n153 = Add(x=w288, y=w287) -> (x+y=w275:dbl)
        "Numeric" <- w275
        n154 = Greater?(x=w275, y=w276) -> (0:w286:bool)
        n155 = And(x=w294, y=w293) -> (x .and. y?=w285:bool)
        n156 = And(x=w285, y=w286) -> (x .and. y?=w284:bool)
        "近标靶是否合格" <- w284
        n157 = case shown="False" w284 {
          tunnel: [w297 w304] -> w292
          tunnel: w291 -> [w298 w304]
          frame False {
            n158 = call "Display Message to User8"() -> ("重测"=w299:bool)  [unwired: 10 in, 1 out]
            n159 = case shown="True" w299 {
              tunnel: w298 -> [w300 w303]
              tunnel: [w300 w301] -> w297
              frame False {
              }
              frame True {
                n160 = call "Push State.vi"("State Head"="检查近调焦", "States In"=w303) -> ("States Out"=w301:string)  [unwired: 13 in]
              }
            }
          }
          frame True {
          }
        }
      }
      frame "检查远调焦" {
        w309 = 0.0
        w311 = 6
        n161 = Unbundle By Name(w330) -> ("Caldata.焦距选择"=w329:T7)
        n162 = call "Display Message to User10"() -> ("error out"=w331:errorcluster)  [unwired: 10 in, 1 out]
        n163 = Add(x=w329, y=3) -> (x+y=w312:u32)
        n164 = Equal?(x=w312, y=w311) -> (x = y?=w323:bool)
        n165 = control-ref of="Array"() -> (w337:refnum<vi>)
        n166 = Equal?(x=w312, y=w311) -> (x = y?=w310:bool)
        n167 = Select(t=0.07, s=w323, f=w309) -> (s? t:f=w321:dbl)
        n168 = Select(t=0.08, s=w310, f=w309) -> (s? t:f=w307:dbl)
        n169 = call "判断调焦.vi"("Arr Refnum"=w337, "选项"=w312, "error in"=w331) -> ("垂直清晰度-数值"=w327:dbl, "垂直清晰度"=w335:bool, "水平清晰度-数值"=w326:dbl, "水平清晰度"=w334:bool)  [unwired: 8 in, 1 out]
        "远调焦垂直清晰度" <- w327
        "远调焦水平清晰度" <- w326
        n170 = Add(x=w321, y=0.11) -> (x+y=w319:dbl)
        n171 = property on="Numeric" class="DigNum (strict)"() -> ("Value"=w318:dbl)  [unwired: 2 in, 2 out]
        n172 = Add(x=w327, y=w326) -> (x+y=w317:dbl)
        n173 = And(x=w335, y=w334) -> (x .and. y?=w324:bool)
        n174 = Greater?(x=w317, y=w319) -> (0:w325:bool)
        n175 = Add(x=w317, y=w318) -> (x+y=w316:dbl)
        n176 = Add(x=w307, y=0.17) -> (x+y=w305:dbl)
        n177 = And(x=w324, y=w325) -> (x .and. y?=w314:bool)
        n178 = Greater?(x=w316, y=w305) -> (0:w315:bool)
        n179 = And(x=w314, y=w315) -> (x .and. y?=w313:bool)
        "远标靶是否合格" <- w313
        n180 = case shown="False" w313 {
          tunnel: [w338 w345] -> w333
          tunnel: w332 -> [w339 w345]
          frame False {
            n181 = call "Display Message to User9"() -> ("重测"=w340:bool)  [unwired: 10 in, 1 out]
            n182 = case shown="True" w340 {
              tunnel: w339 -> [w341 w344]
              tunnel: [w341 w342] -> w338
              frame False {
              }
              frame True {
                n183 = call "Push State.vi"("State Head"="检查远调焦", "States In"=w344) -> ("States Out"=w342:string)  [unwired: 13 in]
              }
            }
          }
          frame True {
          }
        }
      }
      frame "检查锅盖竖纹" {
        n184 = call "Display Message to User13"("error in (no error)"=w348) -> ("error out"=w347:errorcluster, "合格"=→"检查锅盖竖纹是否合格":bool)  [unwired: 9 in]
      }
      frame "读取SNPN" {
        n185 = call "INfo_Get.vi"("error in"=w368, "select"=enum16{"fw", "sn", "pn"}."pn") -> ("error out"=w367:errorcluster, "data out"=w357:u8[], "return"=w365:i32)  [unwired: 7 in]
        n186 = Byte Array To String(unsigned byte array=w357) -> (string=w354:string)
        n187 = Equal To 0?(x=w365) -> (x = 0?=w362:bool)
        n188 = local write "PN"(w354) -> ()
        n189 = call "INfo_Get.vi"("error in"=w367, "select"=enum16{"fw", "sn", "pn"}."sn") -> ("error out"=w360:errorcluster, "data out"=w356:u8[], "return"=w364:i32)  [unwired: 7 in]
        n190 = Byte Array To String(unsigned byte array=w356) -> (string=w353:string)
        n191 = Concatenate Strings(w354, "_", w353) -> (w352:string)
        n192 = Equal To 0?(x=w364) -> (x = 0?=w363:bool)
        n193 = local write "二维码信息"(w352) -> ()
        n194 = local write "SN"(w353) -> ()
        n195 = And(x=w363, y=w362) -> (x .and. y?=w361:bool)
        n196 = case shown="True" w361 {
          tunnel: w360 -> [w372 w375]
          tunnel: [w372 w374] -> w359
          tunnel: w355 -> [_ w373]
          tunnel: ["操作失败关闭相机" w373] -> w358
          frame False {
          }
          frame True {
            w378 = "读取SNPN成功" ("state")
            n197 = local read "process"() -> (w377:string)
            n198 = property on="state" class="Str"(error in=w375, "Value"=w378) -> (error out=w376:errorcluster)  [unwired: 1 in, 1 out]
            n199 = call "process.vi"("error in"=w376, "state"=w378, "process in"=w377) -> ("error out"=w374:errorcluster, "process out"=w379:string)  [unwired: 7 in]
            n200 = local write "process"(w379) -> ()
          }
        }
      }
      frame "切换高增益" {
        w399 = "切换高增益" ("state")
        n201 = local read "process"() -> (w398:string)
        n202 = property on="state" class="Str"(error in=w395, "Value"=w399) -> (error out=w397:errorcluster)  [unwired: 1 in, 1 out]
        n203 = call "process.vi"("error in"=w397, "state"=w399, "process in"=w398) -> ("error out"=w394:errorcluster, "process out"=w396:string)  [unwired: 7 in]
        n204 = local write "process"(w396) -> ()
        n205 = property on="出图" class="Bool (strict)"(error in=w394, "Val(Sgnl)"=FALSE) -> (error out=w392:errorcluster)  [unwired: 1 in, 1 out]
        n206 = call "Wait (ms)__ogtk.vi"("error in (no error)"=w392, "milliseconds to wait"=u32 100) -> ("error out"=w388:errorcluster)  [unwired: 8 in, 1 out]
        n207 = call "切换增益.vi"("error in"=w388, "增益"=1) -> ("error out"=w382:errorcluster, "return"=w387:i32)  [unwired: 8 in]
        n208 = Equal To 0?(x=w387) -> (x = 0?=w386:bool)
        n209 = call "读取增益.vi"("error in"=w382) -> ("error out"=w381:errorcluster, "data"=w380:u16)  [unwired: 8 in, 1 out]
        n210 = property on="出图" class="Bool (strict)"(error in=w381, "Val(Sgnl)"=TRUE ("Value (Signaling)")) -> (error out=w385:errorcluster)  [unwired: 1 in, 1 out]
        n211 = local write "当前增益模式"(w380) -> ()
        n212 = call "Wait (ms)__ogtk.vi"("error in (no error)"=w385, "milliseconds to wait"=u32 8000) -> ("error out"=w384:errorcluster)  [unwired: 8 in, 1 out]
        n213 = case shown="True" w386 {
          tunnel: w384 -> [w406 w409]
          tunnel: [w406 w408] -> w402
          tunnel: w401 -> [_ w414]
          tunnel: ["操作失败关闭相机" w414] -> w400
          frame False {
            n214 = local write "切换增益成功"(FALSE) -> ()
          }
          frame True {
            w412 = "切换高增益成功" ("state")
            n215 = local read "process"() -> (w411:string)
            n216 = property on="state" class="Str"(error in=w409, "Value"=w412) -> (error out=w410:errorcluster)  [unwired: 1 in, 1 out]
            n217 = local write "切换增益成功"(TRUE) -> ()
            n218 = call "process.vi"("error in"=w410, "state"=w412, "process in"=w411) -> ("error out"=w408:errorcluster, "process out"=w413:string)  [unwired: 7 in]
            n219 = local write "process"(w413) -> ()
          }
        }
      }
      frame "切换低增益" {
        w437 = "切换低增益" ("state")
        n220 = local read "process"() -> (w436:string)
        n221 = property on="state" class="Str"(error in=w433, "Value"=w437) -> (error out=w435:errorcluster)  [unwired: 1 in, 1 out]
        n222 = call "process.vi"("error in"=w435, "state"=w437, "process in"=w436) -> ("error out"=w432:errorcluster, "process out"=w434:string)  [unwired: 7 in]
        n223 = local write "process"(w434) -> ()
        n224 = property on="出图" class="Bool (strict)"(error in=w432, "Val(Sgnl)"=FALSE) -> (error out=w424:errorcluster)  [unwired: 1 in, 1 out]
        n225 = call "Wait (ms)__ogtk.vi"("error in (no error)"=w424, "milliseconds to wait"=u32 100) -> ("error out"=w418:errorcluster)  [unwired: 8 in, 1 out]
        n226 = call "切换增益.vi"("error in"=w418, "增益"=0) -> ("error out"=w431:errorcluster, "return"=w427:i32)  [unwired: 8 in]
        n227 = call "读取增益.vi"("error in"=w431) -> ("error out"=w422:errorcluster, "data"=w430:u16, "return"=w429:i32)  [unwired: 8 in]
        n228 = local write "当前增益模式"(w430) -> ()
        n229 = Equal To 0?(x=w429) -> (x = 0?=w428:bool)
        n230 = Equal To 0?(x=w427) -> (x = 0?=w426:bool)
        n231 = And(x=w428, y=w426) -> (x .and. y?=w419:bool)
        n232 = property on="出图" class="Bool (strict)"(error in=w422, "Val(Sgnl)"=TRUE ("Value (Signaling)")) -> (error out=w417:errorcluster)  [unwired: 1 in, 1 out]
        n233 = call "Wait (ms)__ogtk.vi"("error in (no error)"=w417, "milliseconds to wait"=u32 8000) -> ("error out"=w416:errorcluster)  [unwired: 8 in, 1 out]
        n234 = case shown="True" w419 {
          tunnel: w416 -> [w444 w447]
          tunnel: [w444 w446] -> w440
          tunnel: w439 -> [_ w452]
          tunnel: ["操作失败关闭相机" w452] -> w438
          frame False {
            n235 = local write "切换增益成功"(FALSE) -> ()
          }
          frame True {
            w450 = "切换低增益成功" ("state")
            n236 = local read "process"() -> (w449:string)
            n237 = property on="state" class="Str"(error in=w447, "Value"=w450) -> (error out=w448:errorcluster)  [unwired: 1 in, 1 out]
            n238 = local write "切换增益成功"(TRUE) -> ()
            n239 = call "process.vi"("error in"=w448, "state"=w450, "process in"=w449) -> ("error out"=w446:errorcluster, "process out"=w451:string)  [unwired: 7 in]
            n240 = local write "process"(w451) -> ()
          }
        }
      }
      frame "关闭自动快门" {
        w462 = "关闭自动快门" ("state")
        n241 = local read "process"() -> (w463:string)
        n242 = property on="state" class="Str"(error in=w460, "Value"=w462) -> (error out=w464:errorcluster)  [unwired: 1 in, 1 out]
        n243 = call "process.vi"("error in"=w464, "state"=w462, "process in"=w463) -> ("error out"=w459:errorcluster, "process out"=w461:string)  [unwired: 7 in]
        n244 = local write "process"(w461) -> ()
        n245 = call "关闭自动快门.vi"("error in"=w459) -> ("error out"=w456:errorcluster, "return"=w458:i32)  [unwired: 9 in]
        n246 = Equal To 0?(x=w458) -> (x = 0?=w457:bool)
        n247 = case shown="True" w457 {
          tunnel: ["操作失败关闭相机" w474] -> w453
          tunnel: w454 -> [_ w474]
          tunnel: w456 -> [w466 w469]
          tunnel: [w466 w468] -> w455
          frame False {
          }
          frame True {
            w472 = "关闭自动快门成功" ("state")
            n248 = local read "process"() -> (w471:string)
            n249 = property on="state" class="Str"(error in=w469, "Value"=w472) -> (error out=w470:errorcluster)  [unwired: 1 in, 1 out]
            n250 = call "process.vi"("error in"=w470, "state"=w472, "process in"=w471) -> ("error out"=w468:errorcluster, "process out"=w473:string)  [unwired: 7 in]
            n251 = local write "process"(w473) -> ()
          }
        }
      }
      frame "打开自动快门" {
        w490 = "打开自动快门" ("state")
        n252 = local read "process"() -> (w491:string)
        n253 = property on="state" class="Str"(error in=w488, "Value"=w490) -> (error out=w492:errorcluster)  [unwired: 1 in, 1 out]
        n254 = call "process.vi"("error in"=w492, "state"=w490, "process in"=w491) -> ("error out"=w487:errorcluster, "process out"=w489:string)  [unwired: 7 in]
        n255 = local write "process"(w489) -> ()
        n256 = Unbundle By Name(w475) -> ("Caldata.快门时间间隔设置"=w476:T8)
        n257 = call "打开自动快门.vi"("error in"=w487) -> ("error out"=w483:errorcluster, "return"=w477:i32)  [unwired: 9 in]
        n258 = call "设置自动快门间隔.vi"("error in"=w483, "时间间隔设置"=w476) -> ("error out"=w482:errorcluster, "return"=w481:i32)  [unwired: 8 in]
        n259 = Equal To 0?(x=w481) -> (x = 0?=w480:bool)
        n260 = Equal To 0?(x=w477) -> (x = 0?=w479:bool)
        n261 = And(x=w479, y=w480) -> (x .and. y?=w478:bool)
        n262 = case shown="True" w478 {
          tunnel: ["操作失败关闭相机" w501] -> w484
          tunnel: w485 -> [_ w501]
          tunnel: w482 -> [w493 w496]
          tunnel: [w493 w495] -> w486
          frame False {
          }
          frame True {
            w499 = "打开自动快门成功" ("state")
            n263 = local read "process"() -> (w498:string)
            n264 = property on="state" class="Str"(error in=w496, "Value"=w499) -> (error out=w497:errorcluster)  [unwired: 1 in, 1 out]
            n265 = call "process.vi"("error in"=w497, "state"=w499, "process in"=w498) -> ("error out"=w495:errorcluster, "process out"=w500:string)  [unwired: 7 in]
            n266 = local write "process"(w500) -> ()
          }
        }
      }
      frame "绑定ID" {
        w512 = "绑定ID" ("state")
        n267 = local read "process"() -> (w513:string)
        n268 = property on="state" class="Str"(error in=w510, "Value"=w512) -> (error out=w514:errorcluster)  [unwired: 1 in, 1 out]
        n269 = call "process.vi"("error in"=w514, "state"=w512, "process in"=w513) -> ("error out"=w509:errorcluster, "process out"=w511:string)  [unwired: 7 in]
        n270 = local write "process"(w511) -> ()
        n271 = call "绑定ID.vi"("error in"=w509) -> ("error out"=w505:errorcluster, "return"=w504:i32)  [unwired: 9 in]
        n272 = Equal To 0?(x=w504) -> (x = 0?=w502:bool)
        n273 = case shown="True" w502 {
          tunnel: ["操作失败关闭相机" w523] -> w506
          tunnel: w507 -> [_ w523]
          tunnel: w505 -> [w515 w518]
          tunnel: [w515 w517] -> w508
          frame False {
          }
          frame True {
            w521 = "绑定ID成功" ("state")
            n274 = local read "process"() -> (w520:string)
            n275 = property on="state" class="Str"(error in=w518, "Value"=w521) -> (error out=w519:errorcluster)  [unwired: 1 in, 1 out]
            n276 = call "process.vi"("error in"=w519, "state"=w521, "process in"=w520) -> ("error out"=w517:errorcluster, "process out"=w522:string)  [unwired: 7 in]
            n277 = local write "process"(w522) -> ()
          }
        }
      }
      frame "写入SN" {
        n278 = disable-structure shown="Enabled" {
          disable-tunnel: w528 -> [w554 w571]
          disable-tunnel: [w553 w571] -> w527
          disable-tunnel: w526 -> [w552 w572]
          disable-tunnel: [w551 w572] -> w525
          frame Disabled {
            w556 = "写入SN" ("state")
            n279 = Get Date/Time In Seconds() -> (seconds since 1Jan1904=w545:timestamp)
            n280 = Format Date/Time String(time format string (%c)="%d", seconds (now)=w545) -> (date/time string=w541:string)  [unwired: 1 in]
            n281 = Format Date/Time String(time format string (%c)="%Y", seconds (now)=w545) -> (date/time string=w542:string)  [unwired: 1 in]
            n282 = Format Date/Time String(time format string (%c)="%m", seconds (now)=w545) -> (date/time string=w534:string)  [unwired: 1 in]
            n283 = local read "process"() -> (w557:string)
            n284 = Decimal String To Number(string=w541) -> (number=w540:i32)  [unwired: 2 in, 1 out]
            n285 = Decimal String To Number(string=w534) -> (number=w533:i32)  [unwired: 2 in, 1 out]
            n286 = property on="state" class="Str"(error in=w554, "Value"=w556) -> (error out=w558:errorcluster)  [unwired: 1 in, 1 out]
            n287 = Add(x=w540, y=30) -> (x+y=w538:i32)
            n288 = Greater?(x=w533, y=9) -> (0:w535:bool)
            n289 = call "process.vi"("error in"=w558, "state"=w556, "process in"=w557) -> ("error out"=w549:errorcluster, "process out"=w555:string)  [unwired: 7 in]
            n290 = case shown="12" w533 {
              tunnel: ["0A" ("time format string (%c)") "0B" ("time format string (%c)") "0C" ("time format string (%c)")] -> w532
              frame 10, Default {
              }
              frame 11 {
              }
              frame 12 {
              }
            }
            n291 = local write "process"(w555) -> ()
            n292 = Number To Decimal String(number=w538) -> (decimal integer string=w537:string)  [unwired: 1 in]
            n293 = Select(t=w532, s=w535, f=w534) -> (s? t:f=w531:string)
            n294 = local read "当前流水号"() -> (w529:string)
            n295 = Concatenate Strings(w542, w531, w537) -> (w530:string)
            n296 = call "新写入SN.vi"("日期"=w530, "流水号"=w529, "error in"=w549) -> ("return"=w548:i32, "error out"=w547:errorcluster)  [unwired: 11 in]
            n297 = Equal To 0?(x=w548) -> (x = 0?=w550:bool)
            n298 = case shown="True" w550 {
              tunnel: ["操作失败关闭相机" w570] -> w551
              tunnel: w552 -> [_ w570]
              tunnel: w547 -> [w562 w565]
              tunnel: [w562 w564] -> w553
              frame False {
              }
              frame True {
                w568 = "写入SN成功" ("state")
                n299 = local read "process"() -> (w567:string)
                n300 = property on="state" class="Str"(error in=w565, "Value"=w568) -> (error out=w566:errorcluster)  [unwired: 1 in, 1 out]
                n301 = call "process.vi"("error in"=w566, "state"=w568, "process in"=w567) -> ("error out"=w564:errorcluster, "process out"=w569:string)  [unwired: 7 in]
                n302 = local write "process"(w569) -> ()
              }
            }
          }
          frame Enabled {
          }
        }
      }
      frame "写入PN" {
        n303 = disable-structure shown="Enabled" {
          disable-tunnel: w577 -> [w601 w615]
          disable-tunnel: [w600 w615] -> w576
          disable-tunnel: w575 -> [w599 w616]
          disable-tunnel: [w598 w616] -> w574
          disable-tunnel: w573 -> [w596 _]
          frame Disabled {
            w603 = "写入PN" ("state")
            n304 = Unbundle By Name(w596) -> ("Caldata"=w595:T3)
            n305 = Unbundle By Name(w595) -> ("测温功能"=w580:string, "产品名"=w584:string, "分辨率"=w594:string, "镜头"=w582:string, "增益模式"=w590:enum16{"高低增益切换", "高增益"}, "产品料号"=w579:string)
            n306 = local read "process"() -> (w604:string)
            n307 = property on="state" class="Str"(error in=w601, "Value"=w603) -> (error out=w605:errorcluster)  [unwired: 1 in, 1 out]
            n308 = Equal To 0?(x=w590) -> (x = 0?=w591:bool)
            n309 = Select(t="S", s=w591, f="H") -> (s? t:f=w581:string)
            n310 = call "process.vi"("error in"=w605, "state"=w603, "process in"=w604) -> ("error out"=w586:errorcluster, "process out"=w602:string)  [unwired: 7 in]
            n311 = local write "process"(w602) -> ()
            n312 = String Subset(string=w594, offset (0)=0, length (rest)=3 ("length (rest)")) -> (substring=w583:string)
            n313 = call "新写入PN.vi"("产品名"=w584, "测温功能"=w580, "预留（默认XX）"="XX", "分辨率"=w583, "镜头"=w582, "增益模式"=w581, "error in"=w586, "产品料号"=w579) -> ("return"=w585:i32, "error out"=w587:errorcluster)  [unwired: 6 in]
            n314 = Equal To 0?(x=w585) -> (x = 0?=w597:bool)
            n315 = case shown="True" w597 {
              tunnel: ["操作失败关闭相机" w614] -> w598
              tunnel: w599 -> [_ w614]
              tunnel: w587 -> [w606 w609]
              tunnel: [w606 w608] -> w600
              frame False {
              }
              frame True {
                w612 = "写入PN成功" ("state")
                n316 = local read "process"() -> (w611:string)
                n317 = property on="state" class="Str"(error in=w609, "Value"=w612) -> (error out=w610:errorcluster)  [unwired: 1 in, 1 out]
                n318 = call "process.vi"("error in"=w610, "state"=w612, "process in"=w611) -> ("error out"=w608:errorcluster, "process out"=w613:string)  [unwired: 7 in]
                n319 = local write "process"(w613) -> ()
              }
            }
          }
          frame Enabled {
          }
        }
      }
      frame "读取SN" {
        w630 = "读取SN" ("state")
        n320 = local read "process"() -> (w631:string)
        n321 = property on="state" class="Str"(error in=w628, "Value"=w630) -> (error out=w632:errorcluster)  [unwired: 1 in, 1 out]
        n322 = call "process.vi"("error in"=w632, "state"=w630, "process in"=w631) -> ("error out"=w620:errorcluster, "process out"=w629:string)  [unwired: 7 in]
        n323 = local write "process"(w629) -> ()
        n324 = call "INfo_Get.vi"("error in"=w620, "select"=enum16{"fw", "sn", "pn"}."sn") -> ("error out"=w619:errorcluster, "data out"=w618:u8[], "return"=w621:i32)  [unwired: 7 in]
        n325 = Byte Array To String(unsigned byte array=w618) -> (string=w617:string)
        n326 = local write "SN"(w617) -> ()
        n327 = Equal To 0?(x=w621) -> (x = 0?=w623:bool)
        n328 = case shown="True" w623 {
          tunnel: ["操作失败关闭相机" w641] -> w625
          tunnel: w626 -> [_ w641]
          tunnel: w619 -> [w633 w636]
          tunnel: [w633 w635] -> w627
          frame False {
          }
          frame True {
            w639 = "读取SN成功" ("state")
            n329 = local read "process"() -> (w638:string)
            n330 = property on="state" class="Str"(error in=w636, "Value"=w639) -> (error out=w637:errorcluster)  [unwired: 1 in, 1 out]
            n331 = call "process.vi"("error in"=w637, "state"=w639, "process in"=w638) -> ("error out"=w635:errorcluster, "process out"=w640:string)  [unwired: 7 in]
            n332 = local write "process"(w640) -> ()
          }
        }
      }
      frame "读取固件版本" {
        w655 = "读取固件版本" ("state")
        n333 = local read "process"() -> (w656:string)
        n334 = property on="state" class="Str"(error in=w653, "Value"=w655) -> (error out=w657:errorcluster)  [unwired: 1 in, 1 out]
        n335 = call "process.vi"("error in"=w657, "state"=w655, "process in"=w656) -> ("error out"=w645:errorcluster, "process out"=w654:string)  [unwired: 7 in]
        n336 = local write "process"(w654) -> ()
        n337 = call "INfo_Get.vi"("error in"=w645, "select"=enum16{"fw", "sn", "pn"}."fw") -> ("error out"=w644:errorcluster, "data out"=w643:u8[], "return"=w646:i32)  [unwired: 7 in]
        n338 = Byte Array To String(unsigned byte array=w643) -> (string=w642:string)
        n339 = local write "固件版本"(w642) -> ()
        n340 = Equal To 0?(x=w646) -> (x = 0?=w648:bool)
        n341 = case shown="True" w648 {
          tunnel: ["操作失败关闭相机" w666] -> w650
          tunnel: w651 -> [_ w666]
          tunnel: w644 -> [w658 w661]
          tunnel: [w658 w660] -> w652
          frame False {
          }
          frame True {
            w664 = "读取固件版本成功" ("state")
            n342 = local read "process"() -> (w663:string)
            n343 = property on="state" class="Str"(error in=w661, "Value"=w664) -> (error out=w662:errorcluster)  [unwired: 1 in, 1 out]
            n344 = call "process.vi"("error in"=w662, "state"=w664, "process in"=w663) -> ("error out"=w660:errorcluster, "process out"=w665:string)  [unwired: 7 in]
            n345 = local write "process"(w665) -> ()
          }
        }
      }
      frame "计算流水号" {
        w682 = "计算流水号" ("state")
        n346 = local read "process"() -> (w683:string)
        n347 = Unbundle By Name(w677) -> ("Caldata"=w676:T3)
        n348 = property on="state" class="Str"(error in=w680, "Value"=w682) -> (error out=w684:errorcluster)  [unwired: 1 in, 1 out]
        n349 = call "process.vi"("error in"=w684, "state"=w682, "process in"=w683) -> ("error out"=w669:errorcluster, "process out"=w681:string)  [unwired: 7 in]
        n350 = Unbundle By Name(w676) -> ("工位"=w674:string, "产品名"=w670:string)
        n351 = local write "process"(w681) -> ()
        n352 = String Subset(string=w674, offset (0)=4) -> (substring=w671:string)  [unwired: 1 in]
        n353 = call "计算流水号.vi"("功能"=enum16{"流水号归零", "计算流水号"}."计算流水号", "工位"=w671, "产品名"=w670, "error in"=w669) -> ("当前流水号"=→"当前流水号":string, "error out"=w668:errorcluster)  [unwired: 10 in]
        n354 = case shown="No Error" w668 {
          tunnel: [w691 "操作失败关闭相机"] -> w678
          tunnel: w675 -> [w691 _]
          tunnel: w668 -> [w686 w692]
          tunnel: [w685 w692] -> w679
          frame No Error {
            w689 = "计算流水号成功" ("state")
            n355 = local read "process"() -> (w688:string)
            n356 = property on="state" class="Str"(error in=w686, "Value"=w689) -> (error out=w687:errorcluster)  [unwired: 1 in, 1 out]
            n357 = call "process.vi"("error in"=w687, "state"=w689, "process in"=w688) -> ("error out"=w685:errorcluster, "process out"=w690:string)  [unwired: 7 in]
            n358 = local write "process"(w690) -> ()
          }
          frame Error {
          }
        }
      }
      frame "流水号归零" {
        w702 = "流水号归零" ("state")
        n359 = local read "process"() -> (w703:string)
        n360 = Unbundle By Name(w699) -> ("Caldata"=w698:T3)
        n361 = property on="state" class="Str"(error in=w700, "Value"=w702) -> (error out=w704:errorcluster)  [unwired: 1 in, 1 out]
        n362 = call "process.vi"("error in"=w704, "state"=w702, "process in"=w703) -> ("error out"=w695:errorcluster, "process out"=w701:string)  [unwired: 7 in]
        n363 = Unbundle By Name(w698) -> ("产品名"=w696:string)
        n364 = local write "process"(w701) -> ()
        n365 = call "计算流水号.vi"("功能"=enum16{"流水号归零", "计算流水号"}."流水号归零", "产品名"=w696) -> ()  [unwired: 12 in, 2 out]
      }
      frame "打印二维码" {
        n366 = disable-structure shown="Enabled" {
          disable-tunnel: w708 -> [w743 w764]
          disable-tunnel: w707 -> [w734 _]
          disable-tunnel: [w710 w764] -> w705
          frame Disabled {
            w745 = "打印二维码" ("state")
            n367 = local read "二维码信息"() -> (w737:string)
            n368 = local read "process"() -> (w746:string)
            n369 = property on="state" class="Str"(error in=w743, "Value"=w745) -> (error out=w747:errorcluster)  [unwired: 1 in, 1 out]
            n370 = Concatenate Strings("^FDLA,", w737, "^FS") -> (w735:string)
            n371 = call "process.vi"("error in"=w747, "state"=w745, "process in"=w746) -> ("error out"=w741:errorcluster, "process out"=w744:string)  [unwired: 7 in]
            n372 = local write "process"(w744) -> ()
            n373 = local read "物料号"() -> (w715:string)
            n374 = local read "型号"() -> (w717:string)
            n375 = Unbundle By Name(w734) -> ("Caldata.打印机VISA"=w733:refnum<visa-resource-name>)
            n376 = local read "打印列"() -> (w731:u16)
            n377 = Search and Replace String(replace all?=TRUE ("replace all? (F)"), input string="\u0010CT~~CD,~CC^~CT~\n^XA\n~TA000\n~JSN\n^LT0\n^MNW\n^MTT\n^PON\n^PMN\n^LH0,0\n^JMA\n^PR4,4\n~SD25\n^JUS\n^LRN\n^CI27\n^PA0,1,1,0\n^XZ\n^XA\n^MMT\n^PW555\n^LL94\n^LS0\n^FT45,73^BQN,2,2\n^FH\\^FDLA,QWERTYUIOPASDFGHJKLZXCVBNMQWERTYUIOPASDFGHJ^FS\n^FT50,75^A0N,14,15^FH\\^CI28^FDC-76^FS^CI27\n^PQ1,0,1,Y\n^XZ", search string="^FDLA,QWERTYUIOPASDFGHJKLZXCVBNMQWERTYUIOPASDFGHJ^FS", replace string=w735, error in=w741) -> (result string=w721:string, error out=w718:errorcluster)  [unwired: 3 in, 2 out]
            n378 = Concatenate Strings("FH\\^CI28^FD" ("string"), w717, "-", w715, "^FS^CI27" ("string")) -> (w714:string)
            n379 = case shown="4" w731 {
              tunnel: ["^FT45,73^BQN,2,2" "^FT151,73^BQN,2,2" "^FT257,73^BQN,2,2" "^FT363,73^BQN,2,2" "^FT469,73^BQN,2,2"] -> w730
              frame 0, Default {
              }
              frame 1 {
              }
              frame 2 {
              }
              frame 3 {
              }
              frame 4 {
              }
            }
            n380 = Search and Replace String(input string=w721, search string="FH\\^CI28^FDC-76^FS^CI27", replace string=w714, error in=w718) -> (result string=w720:string, error out=w719:errorcluster)  [unwired: 4 in, 2 out]
            n381 = local read "打印列"() -> (w723:u16)
            n382 = Search and Replace String(input string=w720, search string="^FT45,73^BQN,2,2", replace string=w730, error in=w719) -> (result string=w728:string, error out=w727:errorcluster)  [unwired: 4 in, 2 out]
            n383 = case shown="1" w723 {
              tunnel: ["^FT50,75^A0N,14,15^" "^FT156,75^A0N,14,15^" "^FT262,75^A0N,14,15^" "^FT369,75^A0N,14,15^" "^FT475,75^A0N,14,15^"] -> w722
              frame 0, Default {
              }
              frame 1 {
              }
              frame 2 {
              }
              frame 3 {
              }
              frame 4 {
              }
            }
            n384 = Search and Replace String(input string=w728, search string="^FT50,75^A0N,14,15^", replace string=w722, error in=w727) -> (result string=w726:string, error out=w725:errorcluster)  [unwired: 4 in, 2 out]
            n385 = for {
              N: 1 -> [_]
              shift-right: [w752] -> w710
              shift-left: w725 -> [w753]
              shift-right: [w750] -> _
              shift-left: w726 -> [w750]
              shift-right: [w749] -> _
              shift-left: w733 -> [w749]
              shift-right: [w748] -> _
              shift-left: u32 9600 ("波特率") -> [w748]
              n386 = Wait (ms)(milliseconds to wait=u32 200) -> ()  [unwired: 1 out]
              n387 = call "Zebra 串口.vi"("error in"=w753, "write buffer"=w750, "波特率"=w748, "VISA 名称"=w749) -> ("error out"=w752:errorcluster)  [unwired: 7 in]
            }
          }
          frame Enabled {
          }
        }
      }
      frame "生成出厂配置" {
        w773 = "生成出厂配置" ("state")
        n388 = local read "process"() -> (w774:string)
        n389 = property on="state" class="Str"(error in=w771, "Value"=w773) -> (error out=w775:errorcluster)  [unwired: 1 in, 1 out]
        n390 = call "process.vi"("error in"=w775, "state"=w773, "process in"=w774) -> ("error out"=w770:errorcluster, "process out"=w772:string)  [unwired: 7 in]
        n391 = local write "process"(w772) -> ()
        n392 = call "生成出厂配置.vi"("error in"=w770) -> ("error out"=w769:errorcluster, "ture?"=w765:bool)  [unwired: 9 in]
        n393 = case shown="True" w765 {
          tunnel: ["操作失败关闭相机" w785] -> w766
          tunnel: w767 -> [_ w785]
          tunnel: w769 -> [w777 w780]
          tunnel: [w777 w779] -> w768
          frame False {
          }
          frame True {
            w783 = "生成出厂配置成功" ("state")
            n394 = local read "process"() -> (w782:string)
            n395 = property on="state" class="Str"(error in=w780, "Value"=w783) -> (error out=w781:errorcluster)  [unwired: 1 in, 1 out]
            n396 = call "process.vi"("error in"=w781, "state"=w783, "process in"=w782) -> ("error out"=w779:errorcluster, "process out"=w784:string)  [unwired: 7 in]
            n397 = local write "process"(w784) -> ()
          }
        }
      }
      frame "检查模组高增益参数" {
        w813 = u16 4048 ("y")
        w834 = u32[] [2402, 2402, 2402, 2402, 16384, 16384, 48, 48]
        w849 = "检查模组高增益参数" ("state")
        n398 = local read "参数存储地址"() -> (w842:path)
        n399 = local read "ID"() -> (w841:string)
        n400 = local read "process"() -> (w850:string)
        n401 = property on="state" class="Str"(error in=w847, "Value"=w849) -> (error out=w851:errorcluster)  [unwired: 1 in, 1 out]
        n402 = Build Path(base path=w842, name or relative path=w841) -> (appended path=w840:path)
        n403 = call "process.vi"("error in"=w851, "state"=w849, "process in"=w850) -> ("error out"=w845:errorcluster, "process out"=w848:string)  [unwired: 7 in]
        n404 = local write "process"(w848) -> ()
        n405 = call <vilib>:"Check if File or Folder Exists.vi"("path"=w840) -> ("file or folder exists?"=w839:bool, "dup path"=w838:path)  [unwired: 8 in, 1 out]
        n406 = Divide(x=w834, y=2) -> (x/y=w833:dbl[])
        n407 = case shown="False" w839 {
          tunnel: w838 -> [w867 w868]
          tunnel: [w866 w868] -> w837
          frame False {
            n408 = Create Folder(path (use dialog)=w867) -> (created path=w866:path)  [unwired: 2 in, 2 out]
          }
          frame True {
          }
        }
        n409 = for {
          tunnel: string[] ["g1tpdktaddr", "g1tpdktdefaultsetaddr", "g1tpdbtaddr", "g1tpdbtdefaultsetaddr", "g1tpdnuctaddr", "g1tpdnuctdefaultsetaddr", "g1tpdtempparmaddr", "g1tpdtempparmdefaultsetaddr"] -> [w871] mode=indexing
          tunnel: w834 -> [w872] mode=indexing
          tunnel: w837 -> [w877]
          tunnel: [w870] -> w836 mode=indexing
          n410 = Match Pattern(string=w871, regular expression="addr") -> (before substring=w869:string)  [unwired: 1 in, 3 out]
          n411 = Concatenate Strings(w869, ".bin") -> (w874:string)
          n412 = Build Path(base path=w877, name or relative path=w874) -> (appended path=w873:path)
          n413 = call "2DStrArrayToEle.vi"("Mothed"=enum16{"init", "Get", "Set", "Close"}."Get", "AddrName"=w871) -> ("Address"=w878:u32)  [unwired: 6 in, 3 out]
          n414 = call "I2C_flash_to_data.vi"("Path"=w873, "dwLen"=w872, "dwAddr"=w878) -> ("data out"=w870:u8[])  [unwired: 8 in]
        }
        n415 = To Long Integer(number=w833) -> (32bit integer=w832:i32[])
        n416 = Index Array(array=w836) -> (element #1=w835:u8[], element #2=w831:u8[], element #3=w830:u8[], element #4=w829:u8[], element #5=w828:u8[], element #6=w827:u8[], element #7=w793:u8[], element #8=w792:u8[])  [unwired: 16 in]
        n417 = Index Array(array=w832) -> (element #1=w825:i32, element #2=w824:i32, element #3=w823:i32, element #4=w822:i32, element #5=w821:i32, element #6=w820:i32)  [unwired: 6 in]
        n418 = call "U8 to U16.vi"("次数"=w825, "data in"=w835) -> ("data out"=w799:u16[])  [unwired: 13 in]
        n419 = call "U8 to U16.vi"("次数"=w824, "data in"=w831) -> ("data out"=w798:u16[])  [unwired: 13 in]
        n420 = call "U8 to U16.vi"("次数"=w823, "data in"=w830) -> ("data out"=w819:u16[])  [unwired: 13 in]
        n421 = call "U8 to U16.vi"("次数"=w822, "data in"=w829) -> ("data out"=w818:u16[])  [unwired: 13 in]
        n422 = call "U8 to U16.vi"("次数"=w821, "data in"=w828) -> ("data out"=w795:u16[])  [unwired: 13 in]
        n423 = call "U8 to U16.vi"("次数"=w820, "data in"=w827) -> ("data out"=w794:u16[])  [unwired: 13 in]
        n424 = To Word Integer(number=w819) -> (16bit integer=w797:i16[])
        n425 = To Word Integer(number=w818) -> (16bit integer=w796:i16[])
        n426 = call "KT数据判定.vi"("data in"=w799) -> ("result"=w808:bool)  [unwired: 14 in]
        n427 = call "KT数据判定.vi"("data in"=w798) -> ("result"=w807:bool)  [unwired: 14 in]
        n428 = call "BT数据判定.vi"("data in"=w797) -> ("result"=w806:bool)  [unwired: 14 in]
        n429 = call "BT数据判定.vi"("data in"=w796) -> ("result"=w805:bool)  [unwired: 14 in]
        n430 = call "NUC-T判定.vi"("高低增益对比数据"=w813, "data in"=w795) -> ("result"=w804:bool)  [unwired: 6 in]
        n431 = call "NUC-T判定.vi"("高低增益对比数据"=w813, "data in"=w794) -> ("result"=w803:bool)  [unwired: 6 in]
        n432 = call "TPD数据判定.vi"("data in"=w793) -> ("result"=w802:bool)  [unwired: 14 in]
        n433 = call "TPD数据判定.vi"("data in"=w792) -> ("result"=w801:bool)  [unwired: 14 in]
        n434 = local write "KT"(w799) -> ()
        n435 = local write "KT_Default"(w798) -> ()
        n436 = local write "BT"(w797) -> ()
        n437 = local write "BT_Default"(w796) -> ()
        n438 = local write "NUC-T"(w795) -> ()
        n439 = local write "NUC-T_Default"(w794) -> ()
        n440 = local write "Tempparam"(w793) -> ()
        n441 = local write "Tempparam_Default"(w792) -> ()
        n442 = Equal?(x=w799, y=w798) -> (x = y?=w817:bool[])
        n443 = Equal?(x=w797, y=w796) -> (x = y?=w816:bool[])
        n444 = Equal?(x=w795, y=w794) -> (x = y?=w815:bool[])
        n445 = Equal?(x=w793, y=w792) -> (x = y?=w814:bool[])
        n446 = local write "Tempparm_D合格？"(w801) -> ()
        n447 = local write "KT合格？"(w808) -> ()
        n448 = local write "KT_D合格？"(w807) -> ()
        n449 = local write "BT合格？"(w806) -> ()
        n450 = local write "BT_D合格？"(w805) -> ()
        n451 = local write "NUC-T合格?"(w804) -> ()
        n452 = local write "NUC-T_D合格？"(w803) -> ()
        n453 = local write "Tempparm合格？"(w802) -> ()
        n454 = And Array Elements(Boolean array=w817) -> (logical AND=w812:bool)
        n455 = And Array Elements(Boolean array=w816) -> (logical AND=w811:bool)
        n456 = And Array Elements(Boolean array=w815) -> (logical AND=w810:bool)
        n457 = And Array Elements(Boolean array=w814) -> (logical AND=w809:bool)
        n458 = local write "KT一致性"(w812) -> ()
        n459 = local write "NUC-T一致性"(w811) -> ()
        n460 = local write "BT一致性"(w810) -> ()
        n461 = local write "Tempparm一致性"(w809) -> ()
        n462 = Compound Arithmetic op=AND(w808, w807, w806, w805, w804, w803, w802, w801) -> (w800:bool)
        n463 = Compound Arithmetic op=AND(w812, w811, w810, w809, w800) -> (w787:bool)
        n464 = local write "高增益数据合格？"(w787) -> ()
        n465 = Select(t="模组高增益参数合格" ("state"), s=w787, f="模组高增益参数不合格" ("state")) -> (s? t:f=w789:string)
        n466 = case shown="False" w787 {
          tunnel: [w854 w865] -> w846
          tunnel: w845 -> [w855 w864]
          tunnel: w789 -> [w853 w860]
          tunnel: w788 -> [_ w859]
          tunnel: ["操作失败关闭相机" w859] -> w786
          frame False {
            n467 = local read "process"() -> (w857:string)
            n468 = property on="state" class="Str"(error in=w855, "Value"=w853) -> (error out=w856:errorcluster)  [unwired: 1 in, 1 out]
            n469 = call "process.vi"("error in"=w856, "state"=w853, "process in"=w857) -> ("error out"=w854:errorcluster, "process out"=w858:string)  [unwired: 7 in]
            n470 = local write "process"(w858) -> ()
          }
          frame True {
            n471 = local read "process"() -> (w862:string)
            n472 = property on="state" class="Str"(error in=w864, "Value"=w860) -> (error out=w861:errorcluster)  [unwired: 1 in, 1 out]
            n473 = call "process.vi"("error in"=w861, "state"=w860, "process in"=w862) -> ("error out"=w865:errorcluster, "process out"=w863:string)  [unwired: 7 in]
            n474 = local write "process"(w863) -> ()
          }
        }
      }
      frame "检查模组低增益参数" {
        w910 = u16 4208 ("y")
        w931 = u32[] [2402, 2402, 2402, 2402, 16384, 16384, 48, 48]
        w943 = "检查模组低增益参数" ("state")
        n475 = local read "参数存储地址"() -> (w939:path)
        n476 = local read "ID"() -> (w938:string)
        n477 = local read "process"() -> (w944:string)
        n478 = property on="state" class="Str"(error in=w941, "Value"=w943) -> (error out=w945:errorcluster)  [unwired: 1 in, 1 out]
        n479 = Build Path(base path=w939, name or relative path=w938) -> (appended path=w937:path)
        n480 = call "process.vi"("error in"=w945, "state"=w943, "process in"=w944) -> ("error out"=w884:errorcluster, "process out"=w942:string)  [unwired: 7 in]
        n481 = call <vilib>:"Check if File or Folder Exists.vi"("path"=w937) -> ("file or folder exists?"=w936:bool, "dup path"=w935:path)  [unwired: 8 in, 1 out]
        n482 = local write "process"(w942) -> ()
        n483 = Divide(x=w931, y=2) -> (x/y=w930:dbl[])
        n484 = case shown="False" w936 {
          tunnel: w935 -> [w961 w962]
          tunnel: [w960 w962] -> w934
          frame False {
            n485 = Create Folder(path (use dialog)=w961) -> (created path=w960:path)  [unwired: 2 in, 2 out]
          }
          frame True {
          }
        }
        n486 = for {
          tunnel: string[] ["g0tpdktaddr", "g0tpdktdefaultsetaddr", "g0tpdbtaddr", "g0tpdbtdefaultsetaddr", "g0tpdnuctaddr", "g0tpdnuctdefaultsetaddr", "g0tpdtempparmaddr", "g0tpdtempparmdefaultsetaddr"] -> [w965] mode=indexing
          tunnel: w931 -> [w966] mode=indexing
          tunnel: w934 -> [w971]
          tunnel: [w964] -> w933 mode=indexing
          n487 = Match Pattern(string=w965, regular expression="addr") -> (before substring=w963:string)  [unwired: 1 in, 3 out]
          n488 = Concatenate Strings(w963, ".bin") -> (w968:string)
          n489 = Build Path(base path=w971, name or relative path=w968) -> (appended path=w967:path)
          n490 = call "2DStrArrayToEle.vi"("Mothed"=enum16{"init", "Get", "Set", "Close"}."Get", "AddrName"=w965) -> ("Address"=w972:u32)  [unwired: 6 in, 3 out]
          n491 = call "I2C_flash_to_data.vi"("Path"=w967, "dwLen"=w966, "dwAddr"=w972) -> ("data out"=w964:u8[])  [unwired: 8 in]
        }
        n492 = To Long Integer(number=w930) -> (32bit integer=w929:i32[])
        n493 = Index Array(array=w933) -> (element #1=w932:u8[], element #2=w928:u8[], element #3=w927:u8[], element #4=w926:u8[], element #5=w925:u8[], element #6=w924:u8[], element #7=w888:u8[], element #8=w889:u8[])  [unwired: 16 in]
        n494 = Index Array(array=w929) -> (element #1=w922:i32, element #2=w921:i32, element #3=w920:i32, element #4=w919:i32, element #5=w918:i32, element #6=w917:i32)  [unwired: 6 in]
        n495 = call "U8 to U16.vi"("次数"=w922, "data in"=w932) -> ("data out"=w895:u16[])  [unwired: 13 in]
        n496 = call "U8 to U16.vi"("次数"=w921, "data in"=w928) -> ("data out"=w894:u16[])  [unwired: 13 in]
        n497 = call "U8 to U16.vi"("次数"=w920, "data in"=w927) -> ("data out"=w916:u16[])  [unwired: 13 in]
        n498 = call "U8 to U16.vi"("次数"=w919, "data in"=w926) -> ("data out"=w915:u16[])  [unwired: 13 in]
        n499 = call "U8 to U16.vi"("次数"=w918, "data in"=w925) -> ("data out"=w891:u16[])  [unwired: 13 in]
        n500 = call "U8 to U16.vi"("次数"=w917, "data in"=w924) -> ("data out"=w890:u16[])  [unwired: 13 in]
        n501 = To Word Integer(number=w916) -> (16bit integer=w893:i16[])
        n502 = To Word Integer(number=w915) -> (16bit integer=w892:i16[])
        n503 = local write "KT"(w895) -> ()
        n504 = local write "KT_Default"(w894) -> ()
        n505 = local write "BT"(w893) -> ()
        n506 = local write "BT_Default"(w892) -> ()
        n507 = local write "NUC-T"(w891) -> ()
        n508 = local write "NUC-T_Default"(w890) -> ()
        n509 = local write "Tempparam"(w888) -> ()
        n510 = local write "Tempparam_Default"(w889) -> ()
        n511 = call "KT数据判定.vi"("data in"=w895) -> ("result"=w905:bool)  [unwired: 14 in]
        n512 = call "KT数据判定.vi"("data in"=w894) -> ("result"=w904:bool)  [unwired: 14 in]
        n513 = call "BT数据判定.vi"("data in"=w893) -> ("result"=w903:bool)  [unwired: 14 in]
        n514 = call "BT数据判定.vi"("data in"=w892) -> ("result"=w902:bool)  [unwired: 14 in]
        n515 = call "NUC-T判定.vi"("高低增益对比数据"=w910, "data in"=w891) -> ("result"=w901:bool)  [unwired: 6 in]
        n516 = call "NUC-T判定.vi"("高低增益对比数据"=w910, "data in"=w890) -> ("result"=w900:bool)  [unwired: 6 in]
        n517 = call "TPD数据判定.vi"("data in"=w888) -> ("result"=w899:bool)  [unwired: 14 in]
        n518 = call "TPD数据判定.vi"("data in"=w889) -> ("result"=w898:bool)  [unwired: 14 in]
        n519 = Equal?(x=w895, y=w894) -> (x = y?=w914:bool[])
        n520 = Equal?(x=w893, y=w892) -> (x = y?=w913:bool[])
        n521 = Equal?(x=w891, y=w890) -> (x = y?=w912:bool[])
        n522 = Equal?(x=w888, y=w889) -> (x = y?=w911:bool[])
        n523 = local write "Tempparm_D合格？"(w898) -> ()
        n524 = local write "KT合格？"(w905) -> ()
        n525 = local write "KT_D合格？"(w904) -> ()
        n526 = local write "BT合格？"(w903) -> ()
        n527 = local write "BT_D合格？"(w902) -> ()
        n528 = local write "NUC-T合格?"(w901) -> ()
        n529 = local write "NUC-T_D合格？"(w900) -> ()
        n530 = local write "Tempparm合格？"(w899) -> ()
        n531 = And Array Elements(Boolean array=w914) -> (logical AND=w909:bool)
        n532 = And Array Elements(Boolean array=w913) -> (logical AND=w908:bool)
        n533 = And Array Elements(Boolean array=w912) -> (logical AND=w907:bool)
        n534 = And Array Elements(Boolean array=w911) -> (logical AND=w906:bool)
        n535 = local write "KT一致性"(w909) -> ()
        n536 = local write "NUC-T一致性"(w908) -> ()
        n537 = local write "BT一致性"(w907) -> ()
        n538 = local write "Tempparm一致性"(w906) -> ()
        n539 = Compound Arithmetic op=AND(w905, w904, w903, w902, w901, w900, w899, w898) -> (w897:bool)
        n540 = Compound Arithmetic op=AND(w909, w908, w907, w906, w897) -> (w883:bool)
        n541 = local write "低增益数据合格？"(w883) -> ()
        n542 = Select(t="模组高增益参数合格" ("state"), s=w883, f="模组高增益参数不合格" ("state")) -> (s? t:f=w885:string)
        n543 = case shown="True" w883 {
          tunnel: [w948 w959] -> w880
          tunnel: w884 -> [w949 w958]
          tunnel: w885 -> [w947 w954]
          tunnel: w882 -> [_ w953]
          tunnel: ["操作失败关闭相机" w953] -> w881
          frame False {
            n544 = local read "process"() -> (w951:string)
            n545 = property on="state" class="Str"(error in=w949, "Value"=w947) -> (error out=w950:errorcluster)  [unwired: 1 in, 1 out]
            n546 = call "process.vi"("error in"=w950, "state"=w947, "process in"=w951) -> ("error out"=w948:errorcluster, "process out"=w952:string)  [unwired: 7 in]
            n547 = local write "process"(w952) -> ()
          }
          frame True {
            n548 = local read "process"() -> (w956:string)
            n549 = property on="state" class="Str"(error in=w958, "Value"=w954) -> (error out=w955:errorcluster)  [unwired: 1 in, 1 out]
            n550 = call "process.vi"("error in"=w955, "state"=w954, "process in"=w956) -> ("error out"=w959:errorcluster, "process out"=w957:string)  [unwired: 7 in]
            n551 = local write "process"(w957) -> ()
          }
        }
      }
      frame "保存出厂检测数据" {
        w983 = "，" ("string")
        w991 = 3
        w981 = "，" ("string")
        w1035 = i16 3 ("precision (6)")
        w1050 = "生成报表" ("state")
        n552 = Unbundle By Name(w1040) -> ("Caldata.增益模式"=w1037:enum16{"高低增益切换", "高增益"}, "Caldata.操作人"=w1000:string)
        n553 = local read "process"() -> (w1051:string)
        n554 = property on="state" class="Str"(error in=w1048, "Value"=w1050) -> (error out=w1052:errorcluster)  [unwired: 1 in, 1 out]
        n555 = call "process.vi"("error in"=w1052, "state"=w1050, "process in"=w1051) -> ("error out"=w1043:errorcluster, "process out"=w1049:string)  [unwired: 7 in]
        n556 = local read "远标靶是否合格"() -> (w997:bool)
        n557 = case shown="\"高低增益切换\", Default" w1037 {
          tunnel: [w1063 w1068] -> w1016
          tunnel: [w1062 w1068] -> w1013
          tunnel: [w1061 w1068] -> w1010
          tunnel: [w1057 w1068] -> w1005
          tunnel: [w1053 w1068] -> w974
          frame "高低增益切换", Default {
            w1067 = i16 3 ("precision (6)")
            n558 = local read "温度差值2"() -> (w1064:dbl)
            n559 = local read "黑体设定温度2"() -> (w1066:dbl)
            n560 = local read "读取温度2"() -> (w1065:dbl)
            n561 = local read "低增益温度误差在范围内"() -> (w1060:bool)
            n562 = local read "低增益数据合格？"() -> (w1054:bool)
            n563 = Number To Fractional String(number=w1065, precision (6)=w1067) -> (F-format string=w1062:string)  [unwired: 2 in]
            n564 = Number To Fractional String(number=w1064, precision (6)=w1067) -> (F-format string=w1061:string)  [unwired: 2 in]
            n565 = Number To Fractional String(number=w1066, precision (6)=w1067) -> (F-format string=w1063:string)  [unwired: 2 in]
            n566 = Select(t="是", s=w1060, f="否") -> (s? t:f=w1057:string)
            n567 = Select(t="是", s=w1054, f="否") -> (s? t:f=w1053:string)
          }
          frame "高增益" {
            w1068 = "无"
          }
        }
        n568 = local write "process"(w1049) -> ()
        n569 = local read "检查锅盖竖纹是否合格"() -> (w1019:bool)
        n570 = local read "高增益数据合格？"() -> (w976:bool)
        n571 = local read "高增益温度误差在范围内"() -> (w1028:bool)
        n572 = local read "近标靶是否合格"() -> (w1020:bool)
        n573 = local read "盲元合格"() -> (w1025:bool)
        n574 = local read "黑体设定温度1"() -> (w1034:dbl)
        n575 = local read "读取温度1"() -> (w1033:dbl)
        n576 = local read "温度差值1"() -> (w1032:dbl)
        n577 = local read "盲元数"() -> (w1031:dbl)
        n578 = Select(t="是", s=w997, f="否") -> (s? t:f=w993:string)
        n579 = local read "ID"() -> (w1036:string)
        n580 = Get Date/Time In Seconds() -> (seconds since 1Jan1904=w1039:timestamp)
        n581 = Select(t="是", s=w1020, f="否") -> (s? t:f=w994:string)
        n582 = local read "SN"() -> (w1001:string)
        n583 = Format Date/Time String(time format string (%c)="%y/%m/%d/%H/%M", seconds (now)=w1039) -> (date/time string=w999:string)  [unwired: 1 in]
        n584 = Number To Decimal String(number=w1031) -> (decimal integer string=w1004:string)  [unwired: 1 in]
        n585 = Number To Fractional String(number=w1034, precision (6)=w1035) -> (F-format string=w1017:string)  [unwired: 2 in]
        n586 = Number To Fractional String(number=w1033, precision (6)=w1035) -> (F-format string=w1014:string)  [unwired: 2 in]
        n587 = Number To Fractional String(number=w1032, precision (6)=w1035) -> (F-format string=w1011:string)  [unwired: 2 in]
        n588 = Select(t="是", s=w1028, f="否") -> (s? t:f=w1006:string)
        n589 = Select(t="是", s=w1025, f="否") -> (s? t:f=w1003:string)
        n590 = Select(t="是", s=w1019, f="否") -> (s? t:f=w1002:string)
        n591 = Select(t="是", s=w976, f="否") -> (s? t:f=w975:string)
        n592 = local read "二维码信息"() -> (w998:string)
        n593 = Concatenate Strings(w1014, "，" ("string"), w1013) -> (w1008:string)
        n594 = Concatenate Strings(w1011, "，" ("string"), w1010) -> (w1007:string)
        n595 = Concatenate Strings(w1017, "，" ("string"), w1016) -> (w1009:string)
        n596 = local read "固件版本"() -> (w979:string)
        n597 = local read "source path out"() -> (w1041:path)
        n598 = local read "近调焦水平清晰度"() -> (w989:dbl)
        n599 = local read "近调焦垂直清晰度"() -> (w990:dbl)
        n600 = local read "远调焦垂直清晰度"() -> (w988:dbl)
        n601 = local read "远调焦水平清晰度"() -> (w987:dbl)
        n602 = Number To Fractional String(number=w990, precision (6)=w991) -> (F-format string=w986:string)  [unwired: 2 in]
        n603 = Number To Fractional String(number=w988, precision (6)=w991) -> (F-format string=w984:string)  [unwired: 2 in]
        n604 = Number To Fractional String(number=w989, precision (6)=w991) -> (F-format string=w985:string)  [unwired: 2 in]
        n605 = Number To Fractional String(number=w987, precision (6)=w991) -> (F-format string=w982:string)  [unwired: 2 in]
        n606 = Concatenate Strings(w986, w983, w985, w983, w984, w983, w982) -> (w980:string)
        n607 = Concatenate Strings(w994, w981, w993, w981, w980) -> (w992:string)
        n608 = Build Array(w1036, w1009, w1008, w1007, w1006, w1005, w1004, w1003, w992, w1002, w998, w1001, w1000, w979, w974, w975, w999) -> (w1042:string[])
        n609 = call "ExcelSaveData.vi"("error in (no error)"=w1043, "data"=w1042, "template (empty)"=w1041) -> ("error out"=w1044:errorcluster)  [unwired: 8 in]
        n610 = case shown="No Error" w1044 {
          tunnel: [w1075 "生成报表失败，请手动填写报表"] -> w1045
          tunnel: w1046 -> [w1075 _]
          tunnel: [w1070 w1076] -> w1047
          tunnel: w1044 -> [w1069 w1076]
          frame No Error {
            w1073 = "生成报表成功" ("state")
            n611 = local read "process"() -> (w1072:string)
            n612 = property on="state" class="Str"(error in=w1069, "Value"=w1073) -> (error out=w1071:errorcluster)  [unwired: 1 in, 1 out]
            n613 = call "process.vi"("error in"=w1071, "state"=w1073, "process in"=w1072) -> ("error out"=w1070:errorcluster, "process out"=w1074:string)  [unwired: 7 in]
            n614 = local write "process"(w1074) -> ()
          }
          frame Error {
          }
        }
      }
      frame "搬运盲元表到DDR" {
        w1087 = "搬运盲元表到DDR" ("state")
        n615 = local read "process"() -> (w1088:string)
        n616 = property on="state" class="Str"(error in=w1085, "Value"=w1087) -> (error out=w1089:errorcluster)  [unwired: 1 in, 1 out]
        n617 = call "process.vi"("error in"=w1089, "state"=w1087, "process in"=w1088) -> ("error out"=w1084:errorcluster, "process out"=w1086:string)  [unwired: 7 in]
        n618 = local write "process"(w1086) -> ()
        n619 = call "搬运盲元表到DDR.vi"("error in"=w1084) -> ("error out"=w1083:errorcluster, "return"=w1079:i32)  [unwired: 9 in]
        n620 = Equal To 0?(x=w1079) -> (x = 0?=w1078:bool)
        n621 = case shown="True" w1078 {
          tunnel: ["操作失败关闭相机" w1099] -> w1080
          tunnel: w1081 -> [_ w1099]
          tunnel: w1083 -> [w1091 w1094]
          tunnel: [w1091 w1093] -> w1082
          frame False {
          }
          frame True {
            w1097 = "搬运盲元表到DDR成功" ("state")
            n622 = local read "process"() -> (w1096:string)
            n623 = property on="state" class="Str"(error in=w1094, "Value"=w1097) -> (error out=w1095:errorcluster)  [unwired: 1 in, 1 out]
            n624 = call "process.vi"("error in"=w1095, "state"=w1097, "process in"=w1096) -> ("error out"=w1093:errorcluster, "process out"=w1098:string)  [unwired: 7 in]
            n625 = local write "process"(w1098) -> ()
          }
        }
      }
      frame "出厂检完成" {
        w1105 = "出厂检完成" ("state")
        n626 = local read "process"() -> (w1106:string)
        n627 = property on="state" class="Str"(error in=w1103, "Value"=w1105) -> (error out=w1107:errorcluster)  [unwired: 1 in, 1 out]
        n628 = call "process.vi"("error in"=w1107, "state"=w1105, "process in"=w1106) -> ("error out"=w1100:errorcluster, "process out"=w1104:string)  [unwired: 7 in]
        n629 = local write "process"(w1104) -> ()
        n630 = call "Display Message to User2"("error in (no error)"=w1100) -> ("error out"=w1101:errorcluster)  [unwired: 9 in, 1 out]
      }
      frame "保存数据" {
        w1118 = "保存数据" ("state")
        n631 = local read "process"() -> (w1119:string)
        n632 = property on="state" class="Str"(error in=w1116, "Value"=w1118) -> (error out=w1120:errorcluster)  [unwired: 1 in, 1 out]
        n633 = call "process.vi"("error in"=w1120, "state"=w1118, "process in"=w1119) -> ("error out"=w1115:errorcluster, "process out"=w1117:string)  [unwired: 7 in]
        n634 = local write "process"(w1117) -> ()
        n635 = call "保存图像数据.vi"("error in"=w1115) -> ("error out"=w1112:errorcluster, "return"=w1114:i32)  [unwired: 9 in]
        n636 = Equal To 0?(x=w1114) -> (x = 0?=w1113:bool)
        n637 = case shown="True" w1113 {
          tunnel: ["操作失败关闭相机" w1130] -> w1109
          tunnel: w1110 -> [_ w1130]
          tunnel: w1112 -> [w1122 w1125]
          tunnel: [w1122 w1124] -> w1111
          frame False {
          }
          frame True {
            w1128 = "保存数据成功" ("state")
            n638 = local read "process"() -> (w1127:string)
            n639 = property on="state" class="Str"(error in=w1125, "Value"=w1128) -> (error out=w1126:errorcluster)  [unwired: 1 in, 1 out]
            n640 = call "process.vi"("error in"=w1126, "state"=w1128, "process in"=w1127) -> ("error out"=w1124:errorcluster, "process out"=w1129:string)  [unwired: 7 in]
            n641 = local write "process"(w1129) -> ()
          }
        }
      }
      frame "读取盲元数" {
        w1148 = "读取盲元数" ("state")
        n642 = local read "process"() -> (w1149:string)
        n643 = property on="state" class="Str"(error in=w1146, "Value"=w1148) -> (error out=w1150:errorcluster)  [unwired: 1 in, 1 out]
        n644 = call "process.vi"("error in"=w1150, "state"=w1148, "process in"=w1149) -> ("error out"=w1144:errorcluster, "process out"=w1147:string)  [unwired: 7 in]
        n645 = local write "process"(w1147) -> ()
        n646 = call "Display Message to User3"("error in (no error)"=w1144) -> ("error out"=w1134:errorcluster)  [unwired: 9 in, 1 out]
        n647 = Unbundle By Name(w1139) -> ("Caldata.盲元阈值"=w1138:dbl)
        n648 = property on="Intensity Graph" class="IntGraph (strict)"(error in=w1134) -> (error out=w1133:errorcluster, "Value"=w1137:u16[][])  [unwired: 1 in, 1 out]
        n649 = Divide(x=w1137, y=4) -> (x/y=w1135:dbl[][])
        n650 = call "邻域去盲元-子VI.vi"("error in"=w1133, "输入"=w1135, "阈值"=w1138, "尺寸"=3) -> ("盲元表"=w1143:dbl[][], "error out"=w1141:errorcluster)  [unwired: 5 in, 1 out]
        n651 = Add Array Elements(numeric array=w1143) -> (sum=w1131:dbl)
        "盲元数" <- w1131
        n652 = Equal To 0?(x=w1131) -> (x = 0?=w1132:bool)
        n653 = local write "盲元合格"(w1132) -> ()
        n654 = flat-sequence {
          tunnel: w1141 -> [w1152]
          tunnel: [w1151] -> w1140
          frame #0 {
            w1155 = "测试完成" ("state")
            n655 = local read "process"() -> (w1154:string)
            n656 = property on="state" class="Str"(error in=w1152, "Value"=w1155) -> (error out=w1153:errorcluster)  [unwired: 1 in, 1 out]
            n657 = call "process.vi"("error in"=w1153, "state"=w1155, "process in"=w1154) -> ("error out"=w1151:errorcluster, "process out"=w1156:string)  [unwired: 7 in]
            n658 = local write "process"(w1156) -> ()
          }
        }
      }
      frame "盲元标定" {
        w1175 = "盲元标定" ("state")
        n659 = local read "process"() -> (w1176:string)
        n660 = property on="state" class="Str"(error in=w1173, "Value"=w1175) -> (error out=w1177:errorcluster)  [unwired: 1 in, 1 out]
        n661 = call "process.vi"("error in"=w1177, "state"=w1175, "process in"=w1176) -> ("error out"=w1162:errorcluster, "process out"=w1174:string)  [unwired: 7 in]
        n662 = local write "process"(w1174) -> ()
        n663 = Unbundle By Name(w1158) -> ("Caldata.分辨率"=w1157:string)
        n664 = local read "盲元表"() -> (w1163:dbl[][])
        n665 = call "2DStrArrayToEle.vi"("Mothed"=enum16{"init", "Get", "Set", "Close"}."Get", "AddrName"="deadpixaddr") -> ("Address"=w1159:u32)  [unwired: 6 in, 3 out]
        n666 = Add Array Elements(numeric array=w1163) -> (sum=w1164:dbl)
        "标定前盲元" <- w1164
        n667 = Greater?(x=w1164, y=1000.0) -> (0:w1165:bool)
        n668 = Array Size(array=w1163) -> (size(s)=w1172:i32[])
        n669 = Multiply Array Elements(1:w1172) -> (0:w1171:i32)
        n670 = Reshape Array(w1163, w1171) -> (w1170:dbl[])
        n671 = case shown="False" w1165 {
          tunnel: w1170 -> [w1186 _]
          tunnel: w1162 -> [w1185 w1229]
          tunnel: [w1184 w1228] -> w1169
          tunnel: w1168 -> [w1183 _]
          tunnel: [w1182 "读取标定盲元"] -> w1167
          tunnel: w1164 -> [w1181 w1227]
          tunnel: w1159 -> [w1179 _]
          tunnel: w1157 -> [w1178 _]
          frame False {
            n672 = Not Equal To 0?(x=w1181) -> (x != 0?=w1180:bool)
            n673 = case shown="True" w1180 {
              tunnel: w1186 -> [_ w1200]
              tunnel: w1185 -> [w1189 w1198]
              tunnel: [w1188 w1208] -> w1184
              tunnel: w1183 -> [_ w1207]
              tunnel: ["读取标定盲元" w1206] -> w1182
              tunnel: w1179 -> [_ w1194]
              tunnel: w1178 -> [_ w1196]
              frame False {
                w1192 = "盲元为零，无需标定" ("state")
                n674 = local read "process"() -> (w1191:string)
                n675 = property on="state" class="Str"(error in=w1189, "Value"=w1192) -> (error out=w1190:errorcluster)  [unwired: 1 in, 1 out]
                n676 = call "process.vi"("error in"=w1190, "state"=w1192, "process in"=w1191) -> ("error out"=w1188:errorcluster, "process out"=w1193:string)  [unwired: 7 in]
                n677 = local write "process"(w1193) -> ()
              }
              frame True {
                n678 = call "合并盲元.vi"("error in"=w1198, "分辨率"=w1196, "盲元数组"=w1200, "地址"=w1194) -> ("error out"=w1197:errorcluster, "输出盲元数组"=w1199:i32[])  [unwired: 6 in]
                n679 = for {
                  tunnel: w1199 -> [w1225] mode=indexing
                  tunnel: [w1221] -> w1211 mode=indexing
                  n680 = Equal To 0?(x=w1225) -> (x = 0?=w1224:bool)
                  n681 = Select(t=u8 1, s=w1224, f=u8 0) -> (s? t:f=w1221:u8)
                }
                n682 = call "擦除盲元表.vi"("error in"=w1197, "分辨率"=w1196, "address"=w1194) -> ("error out"=w1210:errorcluster, "return"=w1205:i32)  [unwired: 7 in]
                n683 = call "cal8bit.vi"("分辨率"=w1196, "Array"=w1211) -> ("ArrayOut"=w1195:u8[])  [unwired: 9 in]
                n684 = Equal To 0?(x=w1205) -> (x = 0?=w1204:bool)
                n685 = call "写盲元表到flash.vi"("error in"=w1210, "data"=w1195, "dwAddr"=w1194, "分辨率"=w1196) -> ("error out"=w1209:errorcluster, "return"=w1203:i32)  [unwired: 6 in]
                n686 = Equal To 0?(x=w1203) -> (x = 0?=w1202:bool)
                n687 = And(x=w1204, y=w1202) -> (x .and. y?=w1201:bool)
                n688 = case shown="True" w1201 {
                  tunnel: ["操作失败关闭相机" w1220] -> w1206
                  tunnel: w1207 -> [_ w1220]
                  tunnel: w1209 -> [w1212 w1214]
                  tunnel: [w1212 w1215] -> w1208
                  frame False {
                  }
                  frame True {
                    w1218 = "盲元标定成功" ("state")
                    n689 = local read "process"() -> (w1217:string)
                    n690 = property on="state" class="Str"(error in=w1214, "Value"=w1218) -> (error out=w1216:errorcluster)  [unwired: 1 in, 1 out]
                    n691 = call "process.vi"("error in"=w1216, "state"=w1218, "process in"=w1217) -> ("error out"=w1215:errorcluster, "process out"=w1219:string)  [unwired: 7 in]
                    n692 = local write "process"(w1219) -> ()
                  }
                }
              }
            }
          }
          frame True {
            w1232 = "盲元过多，放弃标定" ("state")
            n693 = local write "盲元合格"(FALSE ("盲元标定成功")) -> ()
            n694 = local write "盲元数"(w1227) -> ()
            n695 = local read "process"() -> (w1231:string)
            n696 = property on="state" class="Str"(error in=w1229, "Value"=w1232) -> (error out=w1230:errorcluster)  [unwired: 1 in, 1 out]
            n697 = call "process.vi"("error in"=w1230, "state"=w1232, "process in"=w1231) -> ("error out"=w1228:errorcluster, "process out"=w1233:string)  [unwired: 7 in]
            n698 = local write "process"(w1233) -> ()
          }
        }
      }
      frame "读取标定盲元" {
        w1250 = "读取标定盲元" ("state")
        n699 = local read "process"() -> (w1251:string)
        n700 = property on="state" class="Str"(error in=w1248, "Value"=w1250) -> (error out=w1252:errorcluster)  [unwired: 1 in, 1 out]
        n701 = call "process.vi"("error in"=w1252, "state"=w1250, "process in"=w1251) -> ("error out"=w1247:errorcluster, "process out"=w1249:string)  [unwired: 7 in]
        n702 = Unbundle By Name(w1242) -> ("Caldata.盲元阈值"=w1241:dbl, "Caldata.盲元采样帧数"=w1238:u16)
        n703 = local write "process"(w1249) -> ()
        n704 = call "Display Message to User4"("error in (no error)"=w1247) -> ("error out"=w1240:errorcluster)  [unwired: 9 in, 1 out]
        n705 = for {
          N: w1238 -> [_]
          tunnel: w1241 -> [w1264]
          tunnel: w1240 -> [w1263]
          tunnel: [w1265] -> w1235
          shift-right: [w1253] -> w1237
          shift-left: dbl[][] array192x256[49152 elements] -> [w1258]
          tunnel: [w1257] -> w1236
          n706 = property on="Intensity Graph" class="IntGraph (strict)"(error in=w1263) -> (error out=w1262:errorcluster, "Value"=w1261:u16[][])  [unwired: 1 in, 1 out]
          n707 = Divide(x=w1261, y=4) -> (x/y=w1259:dbl[][])
          n708 = Wait (ms)(milliseconds to wait=200) -> ()  [unwired: 1 out]
          n709 = call "邻域去盲元-子VI.vi"("error in"=w1262, "输入"=w1259, "阈值"=w1264, "尺寸"=3) -> ("盲元表"=w1255:dbl[][], "error out"=w1265:errorcluster)  [unwired: 5 in, 1 out]
          n710 = Add(x=w1255, y=w1258) -> (x+y=w1254:dbl[][])
          n711 = for {
            tunnel: w1254 -> [w1268] mode=indexing
            tunnel: [w1267] -> w1253 mode=indexing
            n712 = for {
              tunnel: w1268 -> [w1270] mode=indexing
              tunnel: [w1269] -> w1267 mode=indexing
              n713 = Greater Or Equal?(x=w1270, y=1.0) -> (x >= y?=w1272:bool)
              n714 = Select(t=1.0, s=w1272, f=w1270) -> (s? t:f=w1269:dbl)
            }
          }
          n715 = Add Array Elements(numeric array=w1253) -> (sum=w1257:dbl)
          n716 = local write "盲元数"(w1257) -> ()
        }
        "盲元表" <- w1237
        n717 = Equal To 0?(x=w1236) -> (x = 0?=w1243:bool)
        "盲元合格" <- w1243
        n718 = case shown="False" w1243 {
          tunnel: [w1274 w1285] -> w1246
          tunnel: w1245 -> [w1276 w1286]
          tunnel: [w1277 w1286] -> w1244
          tunnel: w1235 -> [_ w1285]
          frame False {
            n719 = call "Display Message to User5"() -> ("error out"=w1275:errorcluster, "OK"=w1278:bool)  [unwired: 10 in]
            n720 = case shown="True" w1278 {
              tunnel: [w1280 w1281] -> w1277
              tunnel: w1276 -> [w1280 w1283]
              tunnel: w1275 -> [w1279 w1284]
              tunnel: [w1279 w1284] -> w1274
              frame False {
              }
              frame True {
                n721 = call "Push State.vi"("States In"="盲元标定\n搬运盲元表到DDR\n读取标定盲元", "States End"=w1283) -> ("States Out"=w1281:string)  [unwired: 13 in]
              }
            }
          }
          frame True {
          }
        }
      }
      frame "读取高增益温度" {
        w1307 = "读取温度1" ("state")
        n722 = local read "process"() -> (w1308:string)
        n723 = property on="state" class="Str"(error in=w1305, "Value"=w1307) -> (error out=w1309:errorcluster)  [unwired: 1 in, 1 out]
        n724 = call "process.vi"("error in"=w1309, "state"=w1307, "process in"=w1308) -> ("error out"=w1291:errorcluster, "process out"=w1306:string)  [unwired: 7 in]
        n725 = local write "process"(w1306) -> ()
        n726 = call "Display Message to User7"("error in (no error)"=w1291) -> ("error out"=w1290:errorcluster)  [unwired: 9 in, 1 out]
        n727 = property on="Intensity Graph" class="IntGraph (strict)"() -> ("Cursor.Cursor Position"=w1302:T9)  [unwired: 2 in, 2 out]
        n728 = Unbundle By Name(w1302) -> ("Cursor X"=w1301:dbl, "Cursor Y"=w1300:dbl)
        n729 = Unbundle By Name(w1299) -> ("Caldata.黑体设定温度1"=w1294:dbl, "Caldata.温差范围1"=w1297:dbl)
        "黑体设定温度1" <- w1294
        n730 = call "读取单点温度.vi"("error in"=w1290, "y1"=w1300, "x1"=w1301) -> ("error out"=w1296:errorcluster, "温度"=w1293:dbl)  [unwired: 7 in]
        "读取温度1" <- w1293
        n731 = Subtract(x=w1293, y=w1294) -> (x-y=w1292:dbl)
        "温度差值1" <- w1292
        n732 = Absolute Value(x=w1292) -> (abs(x)=w1298:dbl)
        n733 = Less?(x=w1298, y=w1297) -> (x < y?=w1295:bool)
        "高增益温度误差在范围内" <- w1295
        n734 = case shown="False" w1295 {
          tunnel: w1296 -> [w1315 w1328]
          tunnel: [w1310 w1327] -> w1287
          tunnel: w1304 -> [w1312 w1333]
          tunnel: [w1313 w1333] -> w1303
          frame False {
            n735 = call "Display Message to User6"("error in (no error)"=w1315) -> ("error out"=w1311:errorcluster, "重读"=w1314:bool)  [unwired: 9 in]
            n736 = case shown="True" w1314 {
              tunnel: [w1322 w1323] -> w1313
              tunnel: w1312 -> [w1322 w1324]
              tunnel: w1311 -> [w1317 w1326]
              tunnel: [w1316 w1326] -> w1310
              frame False {
                w1319 = "读取温度完成" ("state")
                n737 = local read "process"() -> (w1320:string)
                n738 = property on="state" class="Str"(error in=w1317, "Value"=w1319) -> (error out=w1321:errorcluster)  [unwired: 1 in, 1 out]
                n739 = call "process.vi"("error in"=w1321, "state"=w1319, "process in"=w1320) -> ("error out"=w1316:errorcluster, "process out"=w1318:string)  [unwired: 7 in]
                n740 = local write "process"(w1318) -> ()
              }
              frame True {
                n741 = call "Push State.vi"("States In"="打快门\n读取高增益温度", "States End"=w1324) -> ("States Out"=w1323:string)  [unwired: 13 in]
              }
            }
          }
          frame True {
            w1330 = "读取温度完成" ("state")
            n742 = local read "process"() -> (w1331:string)
            n743 = property on="state" class="Str"(error in=w1328, "Value"=w1330) -> (error out=w1332:errorcluster)  [unwired: 1 in, 1 out]
            n744 = call "process.vi"("error in"=w1332, "state"=w1330, "process in"=w1331) -> ("error out"=w1327:errorcluster, "process out"=w1329:string)  [unwired: 7 in]
            n745 = local write "process"(w1329) -> ()
          }
        }
        n746 = call "Wait (ms)__ogtk.vi"("error in (no error)"=w1287, "milliseconds to wait"=5000) -> ("error out"=w1288:errorcluster)  [unwired: 8 in, 1 out]
      }
      frame "读取低增益温度" {
        w1354 = "读取温度2" ("state")
        n747 = local read "process"() -> (w1355:string)
        n748 = property on="state" class="Str"(error in=w1352, "Value"=w1354) -> (error out=w1356:errorcluster)  [unwired: 1 in, 1 out]
        n749 = call "process.vi"("error in"=w1356, "state"=w1354, "process in"=w1355) -> ("error out"=w1338:errorcluster, "process out"=w1353:string)  [unwired: 7 in]
        n750 = local write "process"(w1353) -> ()
        n751 = call "Display Message to User15"("error in (no error)"=w1338) -> ("error out"=w1337:errorcluster)  [unwired: 9 in, 1 out]
        n752 = property on="Intensity Graph" class="IntGraph (strict)"() -> ("Cursor.Cursor Position"=w1349:T9)  [unwired: 2 in, 2 out]
        n753 = Unbundle By Name(w1349) -> ("Cursor X"=w1348:dbl, "Cursor Y"=w1347:dbl)
        n754 = Unbundle By Name(w1346) -> ("Caldata.黑体设定温度2"=w1341:dbl, "Caldata.温差范围2"=w1344:dbl)
        "黑体设定温度2" <- w1341
        n755 = call "读取单点温度.vi"("error in"=w1337, "y1"=w1347, "x1"=w1348) -> ("error out"=w1343:errorcluster, "温度"=w1340:dbl)  [unwired: 7 in]
        "读取温度2" <- w1340
        n756 = Subtract(x=w1340, y=w1341) -> (x-y=w1339:dbl)
        "温度差值2" <- w1339
        n757 = Absolute Value(x=w1339) -> (abs(x)=w1345:dbl)
        n758 = Less?(x=w1345, y=w1344) -> (x < y?=w1342:bool)
        "低增益温度误差在范围内" <- w1342
        n759 = case shown="False" w1342 {
          tunnel: w1343 -> [w1362 w1375]
          tunnel: [w1357 w1374] -> w1335
          tunnel: w1351 -> [w1359 w1380]
          tunnel: [w1360 w1380] -> w1350
          frame False {
            n760 = call "Display Message to User14"("error in (no error)"=w1362) -> ("error out"=w1358:errorcluster, "重读"=w1361:bool)  [unwired: 9 in]
            n761 = case shown="True" w1361 {
              tunnel: [w1369 w1370] -> w1360
              tunnel: w1359 -> [w1369 w1371]
              tunnel: w1358 -> [w1364 w1373]
              tunnel: [w1363 w1373] -> w1357
              frame False {
                w1366 = "读取温度完成" ("state")
                n762 = local read "process"() -> (w1367:string)
                n763 = property on="state" class="Str"(error in=w1364, "Value"=w1366) -> (error out=w1368:errorcluster)  [unwired: 1 in, 1 out]
                n764 = call "process.vi"("error in"=w1368, "state"=w1366, "process in"=w1367) -> ("error out"=w1363:errorcluster, "process out"=w1365:string)  [unwired: 7 in]
                n765 = local write "process"(w1365) -> ()
              }
              frame True {
                n766 = call "Push State.vi"("States In"="打快门\n读取低增益温度", "States End"=w1371) -> ("States Out"=w1370:string)  [unwired: 13 in]
              }
            }
          }
          frame True {
            w1377 = "读取温度完成" ("state")
            n767 = local read "process"() -> (w1378:string)
            n768 = property on="state" class="Str"(error in=w1375, "Value"=w1377) -> (error out=w1379:errorcluster)  [unwired: 1 in, 1 out]
            n769 = call "process.vi"("error in"=w1379, "state"=w1377, "process in"=w1378) -> ("error out"=w1374:errorcluster, "process out"=w1376:string)  [unwired: 7 in]
            n770 = local write "process"(w1376) -> ()
          }
        }
        n771 = call "Wait (ms)__ogtk.vi"("error in (no error)"=w1335, "milliseconds to wait"=5000) -> ("error out"=w1334:errorcluster)  [unwired: 8 in, 1 out]
      }
      frame "打快门" {
        w1390 = "打快门" ("state")
        n772 = local read "process"() -> (w1391:string)
        n773 = property on="state" class="Str"(error in=w1388, "Value"=w1390) -> (error out=w1392:errorcluster)  [unwired: 1 in, 1 out]
        n774 = call "process.vi"("error in"=w1392, "state"=w1390, "process in"=w1391) -> ("error out"=w1387:errorcluster, "process out"=w1389:string)  [unwired: 7 in]
        n775 = local write "process"(w1389) -> ()
        n776 = call "打快门.vi"("error in"=w1387) -> ("error out"=w1381:errorcluster, "return"=w1386:i32)  [unwired: 9 in]
        n777 = Equal To 0?(x=w1386) -> (x = 0?=w1385:bool)
        n778 = case shown="True" w1385 {
          tunnel: w1384 -> [_ w1404]
          tunnel: ["操作失败关闭相机" w1404] -> w1383
          tunnel: w1381 -> [w1394 w1399]
          tunnel: [w1394 w1397] -> w1382
          frame False {
          }
          frame True {
            w1401 = "打快门成功" ("state")
            n779 = local read "process"() -> (w1402:string)
            n780 = property on="state" class="Str"(error in=w1399, "Value"=w1401) -> (error out=w1403:errorcluster)  [unwired: 1 in, 1 out]
            n781 = call "process.vi"("error in"=w1403, "state"=w1401, "process in"=w1402) -> ("error out"=w1398:errorcluster, "process out"=w1400:string)  [unwired: 7 in]
            n782 = local write "process"(w1400) -> ()
            n783 = call "Wait (ms)__ogtk.vi"("error in (no error)"=w1398, "milliseconds to wait"=u32 2000) -> ("error out"=w1397:errorcluster)  [unwired: 8 in, 1 out]
          }
        }
      }
      frame "出图到测温等待时间" {
        n784 = Unbundle By Name(w1408) -> ("Caldata.出图到测温等待时间"=w1407:dbl)
        n785 = Multiply(x=w1407, y=1000) -> (x*y=w1405:dbl)
        n786 = call "Wait (ms)__ogtk.vi"("error in (no error)"=w1410, "milliseconds to wait"=w1405) -> ("error out"=w1409:errorcluster)  [unwired: 8 in, 1 out]
      }
      frame "关闭相机" {
        w1421 = "关闭相机" ("state")
        n787 = local read "process"() -> (w1422:string)
        n788 = property on="state" class="Str"(error in=w1419, "Value"=w1421) -> (error out=w1423:errorcluster)  [unwired: 1 in, 1 out]
        n789 = call "process.vi"("error in"=w1423, "state"=w1421, "process in"=w1422) -> ("error out"=w1418:errorcluster, "process out"=w1420:string)  [unwired: 7 in]
        n790 = local write "process"(w1420) -> ()
        n791 = property on="出图" class="Bool (strict)"(error in=w1418, "Val(Sgnl)"=FALSE ("Value (Signaling)")) -> (error out=w1426:errorcluster)  [unwired: 1 in, 1 out]
        n792 = call "Wait (ms)__ogtk.vi"("error in (no error)"=w1426, "milliseconds to wait"=u32 100) -> ("error out"=w1425:errorcluster)  [unwired: 8 in, 1 out]
        n793 = call "Close.vi"("error in"=w1425) -> ("error out"=w1417:errorcluster, "result"=w1416:bool)  [unwired: 9 in]
        n794 = case shown="True" w1416 {
          tunnel: w1414 -> [_ w1436]
          tunnel: ["操作失败关闭相机" w1436] -> w1413
          tunnel: w1417 -> [w1428 w1431]
          tunnel: [w1428 w1430] -> w1415
          frame False {
          }
          frame True {
            w1433 = "关闭相机成功" ("state")
            n795 = local read "process"() -> (w1434:string)
            n796 = property on="state" class="Str"(error in=w1431, "Value"=w1433) -> (error out=w1435:errorcluster)  [unwired: 1 in, 1 out]
            n797 = call "process.vi"("error in"=w1435, "state"=w1433, "process in"=w1434) -> ("error out"=w1430:errorcluster, "process out"=w1432:string)  [unwired: 7 in]
            n798 = local write "process"(w1432) -> ()
          }
        }
      }
      frame "断电重启" {
        w1443 = "断电重启" ("state")
        n799 = local read "process"() -> (w1444:string)
        n800 = property on="state" class="Str"(error in=w1441, "Value"=w1443) -> (error out=w1445:errorcluster)  [unwired: 1 in, 1 out]
        n801 = call "process.vi"("error in"=w1445, "state"=w1443, "process in"=w1444) -> ("error out"=w1439:errorcluster, "process out"=w1442:string)  [unwired: 7 in]
        n802 = local write "process"(w1442) -> ()
        n803 = call "Display Message to User11"("error in (no error)"=w1439) -> ("error out"=w1438:errorcluster)  [unwired: 9 in, 1 out]
      }
      frame "操作失败关闭相机" {
        w1455 = "操作失败关闭相机" ("state")
        n804 = local read "process"() -> (w1456:string)
        n805 = property on="state" class="Str"(error in=w1453, "Value"=w1455) -> (error out=w1457:errorcluster)  [unwired: 1 in, 1 out]
        n806 = call "process.vi"("error in"=w1457, "state"=w1455, "process in"=w1456) -> ("error out"=w1452:errorcluster, "process out"=w1454:string)  [unwired: 7 in]
        n807 = local write "process"(w1454) -> ()
        n808 = property on="出图" class="Bool (strict)"(error in=w1452, "Val(Sgnl)"=FALSE ("Value (Signaling)")) -> (error out=w1460:errorcluster)  [unwired: 1 in, 1 out]
        n809 = call "Wait (ms)__ogtk.vi"("error in (no error)"=w1460, "milliseconds to wait"=u32 100) -> ("error out"=w1459:errorcluster)  [unwired: 8 in, 1 out]
        n810 = call "Close.vi"("error in"=w1459) -> ("error out"=w1450:errorcluster, "result"=w1446:bool)  [unwired: 9 in]
        n811 = case shown="True" w1446 {
          tunnel: w1448 -> [_ w1470]
          tunnel: ["操作失败关闭相机" w1470] -> w1447
          tunnel: w1450 -> [w1462 w1465]
          tunnel: [w1462 w1464] -> w1449
          frame False {
          }
          frame True {
            w1467 = "关闭相机成功" ("state")
            n812 = local read "process"() -> (w1468:string)
            n813 = property on="state" class="Str"(error in=w1465, "Value"=w1467) -> (error out=w1469:errorcluster)  [unwired: 1 in, 1 out]
            n814 = call "process.vi"("error in"=w1469, "state"=w1467, "process in"=w1468) -> ("error out"=w1464:errorcluster, "process out"=w1466:string)  [unwired: 7 in]
            n815 = local write "process"(w1466) -> ()
          }
        }
      }
      frame ">>Exit" {
        n816 = call "P2Judge Queue Management.vi"("Mode"=QueueModeCtl."Destory All", "error in"=w1474) -> ("error out"=w1473:errorcluster)  [unwired: 7 in, 2 out]
      }
      frame ">>Quit" {
        n817 = call "P2Judge Queue Management.vi"("Mode"=QueueModeCtl."Destory", "error in"=w1479, "Queue Index"=w1477) -> ("error out"=w1478:errorcluster)  [unwired: 6 in, 2 out]
      }
    }
    n818 = call <vilib>:"Clear Errors.vi"("error in (no error)"=w12) -> ("error out"=w11:errorcluster)  [unwired: 5 in, 1 out]
  }
  n819 = call "获取版本名字.vi"() -> ("before substring"=→"before substring":string)  [unwired: 11 in]
  n820 = while {
    shift-right: [w1491] -> _
    shift-left: w3 -> [w1493]
    shift-right: [w1483] -> _
    shift-left: _ -> [w1489]
    shift-right: [w1485] -> _
    shift-left: -1 -> [w1486]
    stop <- w1488 stop-if-true
    # "事件处理"
    n821 = call "Pop State.vi"("error in (no error)"=w1489, "Pre States"=w1493) -> ("New State"=w1492:string, "Remaining States"=w1490:string)
    n822 = case shown="\"GetPicture\"" w1492 {
      tunnel: [w1498 w1539 w1545 w1552 w1556 w1561 w1568] -> w1491
      tunnel: w1490 -> [w1497 w1539 w1545 w1552 w1556 w1561 w1568]
      tunnel: [w1501 w1537 w1544 w1553 w1555 w1559 w1564] -> w1484
      tunnel: w1489 -> [w1504 w1538 w1548 w1553 w1555 w1560 w1565]
      tunnel: [_ _ _ _ _ _ TRUE] -> w1488
      tunnel: P2Judge_QueueCtl."Picture" ("Queue Index") -> [w1496 _ _ _ _ _ w1563]
      tunnel: w1486 -> [w1494 w1536 w1547 _ w1554 _ w1562]
      tunnel: [w1495 w1536 w1547 -1 w1554 -1 w1562] -> w1485
      frame "Idle", Default {
        n823 = call "P2Judge Queue Management.vi"("error in"=w1504, "Queue Index"=w1496) -> ("error out"=w1503:errorcluster, "Queue"=w1502:refnum<queue>)  [unwired: 7 in, 1 out]
        n824 = call "Dequeue Element.vi"("error in"=w1503, "time out(ms)"=w1494, "Queue"=w1502) -> ("error out"=w1500:errorcluster, "Command"=w1499:string)  [unwired: 6 in, 1 out]
        n825 = case shown="\"time out\"" w1499 {
          tunnel: [w1507 w1512 w1519 w1522 w1527 w1530 w1535] -> w1501
          tunnel: w1500 -> [w1507 w1512 w1519 w1522 w1527 w1530 w1535]
          tunnel: [w1506 w1510 w1518 w1521 w1524 w1529 w1533] -> w1498
          tunnel: w1497 -> [w1506 w1511 w1518 w1521 w1525 w1529 w1534]
          tunnel: [w1505 w1508 w1514 w1520 -1 w1528 w1531] -> w1495
          tunnel: w1494 -> [w1505 w1508 _ w1520 _ w1528 w1531]
          frame Default {
          }
          frame "time out" {
            n826 = call "Push State.vi"("States In"=w1511, "States End"="GetPicture") -> ("States Out"=w1510:string)  [unwired: 13 in]
          }
          frame "StartPic" {
            n827 = local read "Caldata.Fps"() -> (w1513:u16)
            n828 = Divide(x=u32 1000, y=w1513) -> (x/y=w1516:dbl)
            n829 = Round Toward +Infinity(x=w1516) -> (ceil(x): smallest int >= x=w1515:dbl)
            n830 = To Long Integer(number=w1515) -> (32bit integer=w1514:i32)
          }
          frame "Start" {
          }
          frame "ShoutdownPic" {
            n831 = call "Push State.vi"("States In"=w1525, "States End"="ReleasePicture") -> ("States Out"=w1524:string)  [unwired: 13 in]
          }
          frame "error" {
          }
          frame "Quit" {
            n832 = call "Push State.vi"("States In"=w1534, "States End"=">>Exit\n>>Quit" ("Remaining States")) -> ("States Out"=w1533:string)  [unwired: 13 in]
          }
        }
      }
      frame "Error Handle" {
        n833 = call <vilib>:"Clear Errors.vi"("error in (no error)"=w1538) -> ("error out"=w1537:errorcluster)  [unwired: 5 in, 1 out]
      }
      frame "GetPicture" {
        n834 = local read "分辨率"() -> (w1541:string)
        n835 = call "解析分辨率.vi"("分辨率"=w1541) -> ("number 2"=w1542:i32, "number"=w1543:i32)  [unwired: 9 in]
        n836 = call "get_image.vi"("error in"=w1548, "height"=w1542, "width"=w1543) -> ("error out"=w1544:errorcluster, "data"=→"Intensity Graph" →"Array":u16[][], "Image"=→"Image":T1)  [unwired: 4 in, 2 out]
      }
      frame "ReleasePicture" {
        n837 = local write "Image"(T1 refnum ("Image")) -> ()
        n838 = local write "Intensity Graph"(u16[][] [] ("Intensity Graph")) -> ()
      }
      frame ">>Init" {
      }
      frame ">>Exit" {
        n839 = call "P2Judge Queue Management.vi"("Mode"=QueueModeCtl."Destory All", "error in"=w1560) -> ("error out"=w1559:errorcluster)  [unwired: 7 in, 2 out]
      }
      frame ">>Quit" {
        n840 = call "P2Judge Queue Management.vi"("Mode"=QueueModeCtl."Destory", "error in"=w1565, "Queue Index"=w1563) -> ("error out"=w1564:errorcluster)  [unwired: 6 in, 2 out]
      }
    }
    n841 = call <vilib>:"Clear Errors.vi"("error in (no error)"=w1484) -> ("error out"=w1483:errorcluster)  [unwired: 5 in, 1 out]
  }
  n842 = call "Push State.vi"("States In"="InitGUI") -> ("States Out"=w8:string)  [unwired: 14 in]
  n843 = while {
    shift-right: [w1575] -> _
    shift-left: w8 -> [w1577]
    shift-right: [w1569] -> _
    shift-left: _ -> [w1573]
    stop <- w1572 stop-if-true
    # "事件处理"
    n844 = call "Pop State.vi"("error in (no error)"=w1573, "Pre States"=w1577) -> ("New State"=w1576:string, "Remaining States"=w1574:string)
    n845 = case shown="\"InitGUI\"" w1576 {
      tunnel: [w1580 w1664 w1673 w1674 w1679 w1689 w1693 w1703 w1709 w1715 w1721 w1727 w1733 w1739 w1745 w1751 w1757 w1763 w1769 w1774 w1780] -> w1575
      tunnel: w1574 -> [w1579 w1664 w1673 w1674 w1679 w1689 w1693 w1703 w1709 w1715 w1721 w1727 w1733 w1739 w1745 w1751 w1757 w1763 w1769 w1774 w1780]
      tunnel: [w1583 w1662 w1672 w1675 w1680 w1690 w1694 w1704 w1710 w1716 w1722 w1728 w1734 w1740 w1746 w1752 w1758 w1764 w1768 w1770 w1776] -> w1570
      tunnel: w1573 -> [w1586 w1663 w1672 w1676 w1681 w1691 w1700 w1706 w1712 w1718 w1724 w1730 w1736 w1742 w1748 w1754 w1760 w1766 w1768 w1771 w1777]
      tunnel: [_ _ _ _ _ _ _ _ _ _ _ _ _ _ _ _ _ _ _ _ TRUE] -> w1572
      tunnel: P2Judge_QueueCtl."Main" ("Queue Index") -> [w1578 _ _ _ _ _ _ _ _ _ _ _ _ _ _ _ _ _ _ _ w1775]
      frame "Idle", Default {
        n846 = call "P2Judge Queue Management.vi"("error in"=w1586, "Queue Index"=w1578) -> ("error out"=w1585:errorcluster, "Queue"=w1584:refnum<queue>)  [unwired: 7 in, 1 out]
        n847 = call "Dequeue Element.vi"("error in"=w1585, "Queue"=w1584) -> ("error out"=w1582:errorcluster, "Command"=w1581:string)  [unwired: 7 in, 1 out]
        n848 = case shown="\"流水号归零\"" w1581 {
          tunnel: [w1587 w1591 w1595 w1599 w1603 w1607 w1611 w1615 w1619 w1623 w1627 w1631 w1633 w1637 w1641 w1645 w1649 w1653 w1657 w1661] -> w1583
          tunnel: w1582 -> [w1587 w1591 w1595 w1599 w1603 w1607 w1611 w1615 w1619 w1623 w1627 w1631 w1633 w1637 w1641 w1645 w1649 w1653 w1657 w1661]
          tunnel: [w1588 w1589 w1593 w1597 w1601 w1605 w1609 w1613 w1617 w1621 w1625 w1629 w1635 w1639 w1643 w1647 w1651 w1652 w1656 w1660] -> w1580
          tunnel: w1579 -> [w1588 w1590 w1594 w1598 w1602 w1606 w1610 w1614 w1618 w1622 w1626 w1630 w1634 w1638 w1642 w1646 w1650 w1652 w1655 w1659]
          frame "Idle", Default {
          }
          frame "time out" {
            n849 = call "Push State.vi"("States In"=w1590) -> ("States Out"=w1589:string)  [unwired: 14 in]
          }
          frame "打快门" {
            n850 = call "Push State.vi"("States In"=w1594, "States End"="打快门") -> ("States Out"=w1593:string)  [unwired: 13 in]
          }
          frame "读ID" {
            n851 = call "Push State.vi"("States In"=w1598, "States End"="读ID") -> ("States Out"=w1597:string)  [unwired: 13 in]
          }
          frame "写入配置" {
            n852 = call "Push State.vi"("States In"=w1602, "States End"="写入配置") -> ("States Out"=w1601:string)  [unwired: 13 in]
          }
          frame "撤销标定" {
            n853 = call "Push State.vi"("States In"=w1606, "States End"="撤销标定") -> ("States Out"=w1605:string)  [unwired: 13 in]
          }
          frame "打开AGC" {
            n854 = call "Push State.vi"("States In"=w1610, "States End"="打开AGC") -> ("States Out"=w1609:string)  [unwired: 13 in]
          }
          frame "读取盲元数" {
            n855 = call "Push State.vi"("States In"=w1614, "States End"="读取盲元数") -> ("States Out"=w1613:string)  [unwired: 13 in]
          }
          frame "完成" {
            n856 = call "Push State.vi"("States In"=w1618, "States End"="完成") -> ("States Out"=w1617:string)  [unwired: 13 in]
          }
          frame "Button - Option" {
            n857 = call "Push State.vi"("States In"=w1622, "States End"=">>WinOption") -> ("States Out"=w1621:string)  [unwired: 13 in]
          }
          frame "Button - Searchdata" {
            n858 = call "Push State.vi"("States In"=w1626, "States End"="Searchdata") -> ("States Out"=w1625:string)  [unwired: 13 in]
          }
          frame "Button - start" {
            n859 = call "Push State.vi"("States In"=w1630, "States End"="Start") -> ("States Out"=w1629:string)  [unwired: 13 in]
          }
          frame "出图" {
            n860 = call "Push State.vi"("States In"=w1634, "States End"="Picture") -> ("States Out"=w1635:string)  [unwired: 13 in]
          }
          frame "打印二维码" {
            n861 = call "Push State.vi"("States In"=w1638, "States End"="打印二维码") -> ("States Out"=w1639:string)  [unwired: 13 in]
          }
          frame "流水号归零" {
            n862 = call "Push State.vi"("States In"=w1642, "States End"="流水号归零") -> ("States Out"=w1643:string)  [unwired: 13 in]
          }
          frame "开始高温采集" {
            n863 = call "Push State.vi"("States In"=w1646, "States End"="开始高温采集") -> ("States Out"=w1647:string)  [unwired: 13 in]
          }
          frame "开始低温采集" {
            n864 = call "Push State.vi"("States In"=w1650, "States End"="开始低温采集") -> ("States Out"=w1651:string)  [unwired: 13 in]
          }
          frame "error" {
          }
          frame "Button - Exit" {
            n865 = call "Push State.vi"("States In"=w1655, "States End"=">>Exit\n>>Quit" ("Remaining States")) -> ("States Out"=w1656:string)  [unwired: 13 in]
          }
          frame "Menu - Exit" {
            n866 = call "Push State.vi"("States In"=w1659, "States End"=">>Exit\n>>Quit" ("Remaining States")) -> ("States Out"=w1660:string)  [unwired: 13 in]
          }
        }
      }
      frame "Error Handle" {
        n867 = call <vilib>:"Clear Errors.vi"("error in (no error)"=w1663) -> ("error out"=w1662:errorcluster)  [unwired: 5 in, 1 out]
      }
      frame "InitGUI" {
        w1665 = FALSE ("Tempparm_D合格？")
        w1666 = 0.0 ("远调焦垂直清晰度")
        w1667 = "" ("state")
        n868 = local write "出图"(FALSE ("出图")) -> ()
        n869 = local write "process"("" ("process")) -> ()
        n870 = local write "二维码信息"(w1667) -> ()
        n871 = local write "state"(w1667) -> ()
        n872 = local write "ID"(w1667) -> ()
        n873 = local write "远调焦垂直清晰度"(w1666) -> ()
        n874 = local write "远调焦水平清晰度"(w1666) -> ()
        n875 = local write "Image"(T1 refnum ("Image")) -> ()
        n876 = local write "Intensity Graph"(u16[][] [] ("Intensity Graph")) -> ()
        n877 = local write "近调焦垂直清晰度"(w1666) -> ()
        n878 = local write "近调焦水平清晰度"(w1666) -> ()
        n879 = local write "Tempparm_D合格？"(w1665) -> ()
        n880 = local write "NUC-T_D合格？"(w1665) -> ()
        n881 = local write "BT_D合格？"(w1665) -> ()
        n882 = local write "KT_D合格？"(w1665) -> ()
        n883 = local write "Tempparm合格？"(w1665) -> ()
        n884 = local write "NUC-T合格?"(w1665) -> ()
        n885 = local write "BT合格？"(w1665) -> ()
        n886 = local write "KT合格？"(w1665) -> ()
        n887 = local write "KT一致性"(w1665) -> ()
        n888 = local write "NUC-T一致性"(w1665) -> ()
        n889 = local write "BT一致性"(w1665) -> ()
        n890 = local write "Tempparm一致性"(w1665) -> ()
        n891 = local write "低增益数据合格？"(w1665) -> ()
        n892 = local write "高增益数据合格？"(w1665) -> ()
      }
      frame ">>WinOption" {
        n893 = call "WinOption.vi"("error in"=w1676) -> ("error out"=w1675:errorcluster)  [unwired: 10 in]
      }
      frame "Searchdata" {
        n894 = call "Path.vi"() -> ("path"=w1678:T6)  [unwired: 9 in]
        n895 = Unbundle By Name(w1678) -> ("Datasave"=w1677:path)
        n896 = call "OpenFile.vi"("error in"=w1681, "路径"=w1677) -> ("error out"=w1680:errorcluster)  [unwired: 9 in]
      }
      frame "Start" {
        w1683 = 0.0 ("盲元数")
        w1682 = "" ("流水号")
        w1684 = FALSE
        w1685 = FALSE ("出图")
        n897 = local write "盲元合格"(w1684) -> ()
        n898 = local write "切换增益成功"(w1684) -> ()
        n899 = local write "温度差值1"(w1683) -> ()
        n900 = local write "读取温度2"(w1683) -> ()
        n901 = local write "读取温度1"(w1683) -> ()
        n902 = local write "盲元数"(w1683) -> ()
        n903 = local write "温度差值2"(w1683) -> ()
        n904 = local write "低增益温度误差在范围内"(w1685) -> ()
        n905 = local write "高增益温度误差在范围内"(w1685) -> ()
        n906 = local write "process"("" ("process")) -> ()
        n907 = local write "出图"(w1685) -> ()
        n908 = local write "state"("" ("state")) -> ()
        n909 = local write "远调焦垂直清晰度"(w1683) -> ()
        n910 = local write "远调焦水平清晰度"(w1683) -> ()
        n911 = local write "远标靶是否合格"(w1684) -> ()
        n912 = local write "近标靶是否合格"(w1684) -> ()
        n913 = local write "固件版本"(w1682) -> ()
        n914 = local write "PN"(w1682) -> ()
        n915 = local write "SN"(w1682) -> ()
        n916 = local write "近调焦垂直清晰度"(w1683) -> ()
        n917 = local write "近调焦水平清晰度"(w1683) -> ()
        n918 = call "P2Judge Queue Management.vi"("Mode"=QueueModeCtl."Send>All", "error in"=w1691, "Command"="Start") -> ("error out"=w1690:errorcluster)  [unwired: 6 in, 2 out]
      }
      frame "Picture" {
        n919 = local read "出图"() -> (w1697:bool)
        n920 = Select(t="StartPic" ("Command"), s=w1697, f="ShoutdownPic") -> (s? t:f=w1695:string)
        n921 = call "P2Judge Queue Management.vi"("Mode"=QueueModeCtl."Send", "error in"=w1700, "Command"=w1695, "Queue Index"=P2Judge_QueueCtl."Picture") -> ("error out"=w1694:errorcluster)  [unwired: 5 in, 2 out]
      }
      frame "开始高温采集" {
        n922 = call "P2Judge Queue Management.vi"("Mode"=QueueModeCtl."Send", "error in"=w1706, "Command"="开始高温采集", "Queue Index"=P2Judge_QueueCtl."Picture") -> ("error out"=w1704:errorcluster)  [unwired: 5 in, 2 out]
      }
      frame "开始低温采集" {
        n923 = call "P2Judge Queue Management.vi"("Mode"=QueueModeCtl."Send", "error in"=w1712, "Command"="开始低温采集", "Queue Index"=P2Judge_QueueCtl."Picture") -> ("error out"=w1710:errorcluster)  [unwired: 5 in, 2 out]
      }
      frame "打快门" {
        n924 = call "P2Judge Queue Management.vi"("Mode"=QueueModeCtl."Send", "error in"=w1718, "Command"="打快门", "Queue Index"=P2Judge_QueueCtl."Device") -> ("error out"=w1716:errorcluster)  [unwired: 5 in, 2 out]
      }
      frame "读ID" {
        n925 = call "P2Judge Queue Management.vi"("Mode"=QueueModeCtl."Send", "error in"=w1724, "Command"="读ID", "Queue Index"=P2Judge_QueueCtl."Device") -> ("error out"=w1722:errorcluster)  [unwired: 5 in, 2 out]
      }
      frame "写入配置" {
        n926 = call "P2Judge Queue Management.vi"("Mode"=QueueModeCtl."Send", "error in"=w1730, "Command"="写入配置", "Queue Index"=P2Judge_QueueCtl."Device") -> ("error out"=w1728:errorcluster)  [unwired: 5 in, 2 out]
      }
      frame "打印二维码" {
        n927 = call "P2Judge Queue Management.vi"("Mode"=QueueModeCtl."Send", "error in"=w1736, "Command"="打印二维码", "Queue Index"=P2Judge_QueueCtl."Device") -> ("error out"=w1734:errorcluster)  [unwired: 5 in, 2 out]
      }
      frame "流水号归零" {
        n928 = call "P2Judge Queue Management.vi"("Mode"=QueueModeCtl."Send", "error in"=w1742, "Command"="流水号归零", "Queue Index"=P2Judge_QueueCtl."Device") -> ("error out"=w1740:errorcluster)  [unwired: 5 in, 2 out]
      }
      frame "撤销标定" {
        n929 = call "P2Judge Queue Management.vi"("Mode"=QueueModeCtl."Send", "error in"=w1748, "Command"="撤销标定", "Queue Index"=P2Judge_QueueCtl."Device") -> ("error out"=w1746:errorcluster)  [unwired: 5 in, 2 out]
      }
      frame "打开AGC" {
        n930 = call "P2Judge Queue Management.vi"("Mode"=QueueModeCtl."Send", "error in"=w1754, "Command"="打开AGC", "Queue Index"=P2Judge_QueueCtl."Device") -> ("error out"=w1752:errorcluster)  [unwired: 5 in, 2 out]
      }
      frame "读取盲元数" {
        n931 = call "P2Judge Queue Management.vi"("Mode"=QueueModeCtl."Send", "error in"=w1760, "Command"="读取盲元数", "Queue Index"=P2Judge_QueueCtl."Device") -> ("error out"=w1758:errorcluster)  [unwired: 5 in, 2 out]
      }
      frame "完成" {
        n932 = call "P2Judge Queue Management.vi"("Mode"=QueueModeCtl."Send", "error in"=w1766, "Command"="完成", "Queue Index"=P2Judge_QueueCtl."Device") -> ("error out"=w1764:errorcluster)  [unwired: 5 in, 2 out]
      }
      frame ">>Init" {
      }
      frame ">>Exit" {
        n933 = call "P2Judge Queue Management.vi"("Mode"=QueueModeCtl."Send>All", "error in"=w1771, "Command"="Quit") -> ("error out"=w1770:errorcluster)  [unwired: 6 in, 2 out]
      }
      frame ">>Quit" {
        n934 = call "P2Judge Queue Management.vi"("Mode"=QueueModeCtl."Destory", "error in"=w1777, "Queue Index"=w1775) -> ("error out"=w1776:errorcluster)  [unwired: 6 in, 2 out]
      }
    }
    n935 = call <vilib>:"Clear Errors.vi"("error in (no error)"=w1570) -> ("error out"=w1569:errorcluster)  [unwired: 5 in, 1 out]
  }
  n936 = while {
    tunnel: 50 -> [w1784]
    stop <- w1781 stop-if-true
    # "消息捕获"
    n937 = event shown="[0] Timeout" {
      selector: _ -> [_ _ _ _ _]
      dyn-events: _ -> [_ _ _ _ _]
      timeout: w1784 -> [_ _ _ _ _]
      tunnel: P2Judge_QueueCtl."Main" ("Queue Index") -> [_ w1793 w1797 w1800 w1803]
      tunnel: QueueModeCtl."Send" ("Mode") -> [_ w1792 w1796 w1799 w1802]
      tunnel: [w1785 _ _ _ _] -> w1781
      event Timeout {
        n938 = event-data() -> ()  [unwired: 1 in, 3 out]
        n939 = call "P2Judge Queue Management.vi"("Mode"=QueueModeCtl."<no operate>") -> ("Status"=w1786:bool[])  [unwired: 8 in, 2 out]
        n940 = Or Array Elements(Boolean array=w1786) -> (logical OR=w1787:bool)
        n941 = case shown="True" w1787 {
          tunnel: [TRUE _] -> w1785
          frame False {
            n942 = property class="App"() -> ("App.Kind"=w1790:T10)  [unwired: 2 in, 2 out]
            n943 = case shown="\"invalid app kind\", Default" w1790 {
              frame "invalid app kind", Default {
                n944 = Quit LabVIEW(quit? (T)=TRUE ("退出？(T)")) -> ()
              }
              frame "Development System" {
              }
            }
          }
          frame True {
          }
        }
      }
      event Menu Selection (User) {
        n945 = event-data() -> ("ItemTag"=w1794:string)  [unwired: 1 in, 6 out]
        n946 = call "P2Judge Queue Management.vi"("Mode"=w1792, "Command"=w1794, "Queue Index"=w1793) -> ()  [unwired: 6 in, 3 out]
      }
      event "Button - Option", "Button - Searchdata", "Button - start", "出图", "打快门", "读ID", "写入配置", "打开AGC", "读取盲元数", "完成", "Button - Exit": Value Change {
        n947 = event-data() -> ("CtlRef"=w1798:refnum<vi>)  [unwired: 1 in, 5 out]
        n948 = property class="Bool"(reference=w1798) -> ("Label.Text"=w1795:string)  [unwired: 1 in, 2 out]
        n949 = call "P2Judge Queue Management.vi"("Mode"=w1796, "Command"=w1795, "Queue Index"=w1797) -> ()  [unwired: 6 in, 3 out]
      }
      event "手动打印二维码": Value Change {
        n950 = event-data() -> ()  [unwired: 1 in, 6 out]
        n951 = call "P2Judge Queue Management.vi"("Mode"=w1799, "Command"="打印二维码", "Queue Index"=w1800) -> ()  [unwired: 6 in, 3 out]
      }
      event "流水号归零": Value Change {
        n952 = event-data() -> ()  [unwired: 1 in, 6 out]
        n953 = call "P2Judge Queue Management.vi"("Mode"=w1802, "Command"="流水号归零", "Queue Index"=w1803) -> ()  [unwired: 6 in, 3 out]
      }
    }
  }
